vi "Register gRPC Messages.vi"(8 "error in (no error)":errorcluster, 11 "gRPC ID":T1) -> (0 "error out":errorcluster, 3 "gRPC ID Out":T1)   [LabVIEW 2021, in "NI Switch_client.lvlib"]
uses:
  NI Switch_client.lvlib
  <vilib>/gRPC/LabVIEW gRPC Library/Shared/grpcId.ctl
  <vilib>/gRPC/LabVIEW gRPC Library/Server API/typeDefs/Message Metadata.ctl
  <vilib>/gRPC/LabVIEW gRPC Library/Server API/typeDefs/Message Element Metadata.ctl
  <vilib>/gRPC/LabVIEW gRPC Library/Server API/typeDefs/Message Element Type.ctl
  <vilib>/gRPC/LabVIEW gRPC Library/Server API/typeDefs/Enum Metadata.ctl
  <vilib>/gRPC/LabVIEW gRPC Library/grpc-lvsupport-release.lvlib
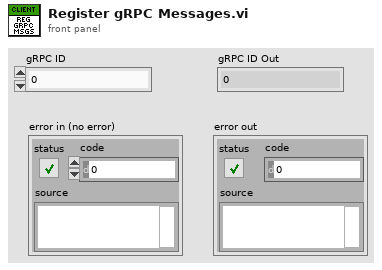
[diagram p1: front panel]
types:
  T1 = typedef "grpc-lvsupport-release.lvlib/grpcId.ctl" = u64
  T2 = typedef "grpc-lvsupport-release.lvlib/Enum Metadata.ctl" = cluster{"Version":i32, "Name":string, "Type Url":string, "Enum Values":string, "Allow Alias":bool}
  T3 = typedef "grpc-lvsupport-release.lvlib/Message Metadata.ctl" = cluster{"Version":i32, "Name":string, "Type Url":string, "Elements":T4[], "Has Oneof":bool}
  T4 = typedef "grpc-lvsupport-release.lvlib/Message Element Metadata.ctl" = cluster{"Field Name":string, "Embedded Message Name":string, "Protobuf Index":i32, "MessageElementType":T5, "Repeated":bool, "Is in Oneof":bool, "Oneof Container Name":string}
  T5 = typedef "grpc-lvsupport-release.lvlib/Message Element Type.ctl" = enum32{"Int32Value", "FloatValue", "DoubleValue", "BoolValue", "StringValue", "MessageValue", "Int64Value", "UInt32Value", "UInt64Value", "EnumValue", "Bytes", "Fixed64", "Fixed32", "SFixed64", "SFixed32", "SInt64", "SInt32"}
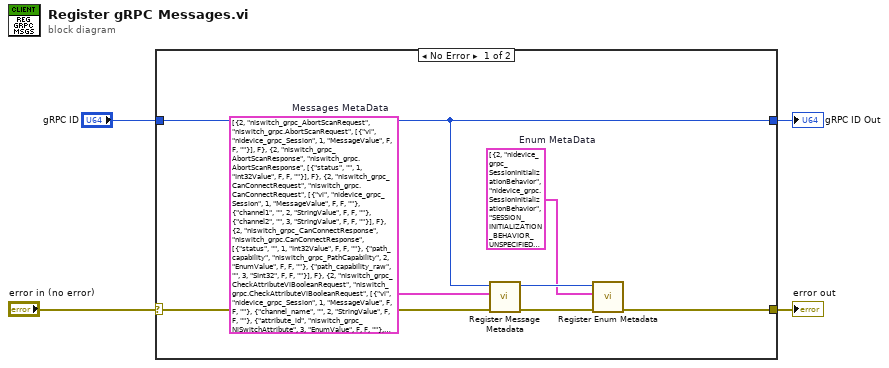
[diagram p0: block diagram]
diagram:
  n1 = case shown="No Error" "error in (no error)" {
    selector: "error in (no error)" -> [w10 w13]
    tunnel: [w9 w12] -> w1
    tunnel: [w6 w13] -> w4
    tunnel: "gRPC ID" -> [w9 w12]
    frame No Error {
      w5 = T2[] [{"Version"=2, "Name"="nidevice_grpc_SessionInitializationBehavior", "Type Url"="nidevice_grpc.SessionInitializationBehavior", "Enum Values"="SESSION_INITIALIZATION_BEHAVIOR_UNSPECIFIED=0;SESSION_INITIALIZATION_BEHAVIOR_INITIALIZE_NEW=1;SESSION_INITIALIZATION_BEHAVIOR_ATTACH_TO_EXISTING=2", "Allow Alias"=FALSE}, {"Version"=2, "Name"="niswitch_grpc_NiSwitchAttribute", "Type Url"="niswitch_grpc.NiSwitchAttribute", "Enum Values"="NISWITCH_ATTRIBUTE_UNSPECIFIED=0;NISWITCH_ATTRIBUTE_RANGE_CHECK=1050002;NISWITCH_ATTRIBUTE_QUERY_INSTRUMENT_STATUS=1050003;NISWITCH_ATTRIBUTE_CACHE=1050004;NISWITCH_ATTRIBUTE_SIMULATE=1050005;NISWITCH_ATTRIBUTE_RECORD_COERCIONS=1050006;NISWITCH_ATTRIBUTE_DRIVER_SETUP=1050007;NISWITCH_ATTRIBUTE_INTERCHANGE_CHECK=1050021;NISWITCH_ATTRIBUTE_CHANNEL_COUNT=1050203;NISWITCH_ATTRIBUTE_SPECIFIC_DRIVER_PREFIX=1050302;NISWITCH_ATTRIBUTE_IO_RESOURCE_DESCRIPTOR=1050304;NISWITCH_ATTRIBUTE_LOGICAL_NAME=1050305;NISWITCH_ATTRIBUTE_SUPPORTED_INSTRUMENT_MODELS=1050327;NISWITCH_ATTRIBUTE_GROUP_CAPABILITIES=1050401;NISWITCH_ATTRIBUTE_INSTRUMENT_FIRMWARE_REVISION=1050510;NISWITCH_ATTRIBUTE_INSTRUMENT_MANUFACTURER=1050511;NISWITCH_ATTRIBUTE_INSTRUMENT_MODEL=1050512;NISWITCH_ATTRIBUTE_SPECIFIC_DRIVER_VENDOR=1050513;NISWITCH_ATTRIBUTE_SPECIFIC_DRIVER_DESCRIPTION=1050514;NISWITCH_ATTRIBUTE_SPECIFIC_DRIVER_CLASS_SPEC_MAJOR_VERSION=1050515;NISWITCH_ATTRIBUTE_SPECIFIC_DRIVER_CLASS_SPEC_MINOR_VERSION=1050516;NISWITCH_ATTRIBUTE_SPECIFIC_DRIVER_REVISION=1050551;NISWITCH_ATTRIBUTE_SERIAL_NUMBER_I32=1150001;NISWITCH_ATTRIBUTE_IS_WAITING_FOR_TRIG=1150004;NISWITCH_ATTRIBUTE_TRIGGER_MODE=1150005;NISWITCH_ATTRIBUTE_MASTER_SLAVE_TRIGGER_BUS=1150006;NISWITCH_ATTRIBUTE_MASTER_SLAVE_SCAN_ADVANCED_BUS=1150007;NISWITCH_ATTRIBUTE_CABLED_MODULE_TRIGGER_BUS=1150008;NISWITCH_ATTRIBUTE_CABLED_MODULE_SCAN_ADVANCED_BUS=1150009;NISWITCH_ATTRIBUTE_TRIGGER_INPUT_POLARITY=1150010;NISWITCH_ATTRIBUTE_SCAN_ADVANCED_POLARITY=1150011;NISWITCH_ATTRIBUTE_PARSED_SCAN_LIST=1150012;NISWITCH_ATTRIBUTE_HANDSHAKING_INITIATION=1150013;NISWITCH_ATTRIBUTE_NUMBER_OF_RELAYS=1150014;NISWITCH_ATTRIBUTE_SERIAL_NUMBER=1150015;NISWITCH_ATTRIBUTE_DIGITAL_FILTER_ENABLE=1150016;NISWITCH_ATTRIBUTE_POWER_DOWN_LATCHING_RELAYS_AFTER_DEBOUNCE=1150017;NISWITCH_ATTRIBUTE_ANALOG_BUS_SHARING_ENABLE=1150018;NISWITCH_ATTRIBUTE_TEMPERATURE=1150019;NISWITCH_ATTRIBUTE_IS_SOURCE_CHANNEL=1250001;NISWITCH_ATTRIBUTE_IS_DEBOUNCED=1250002;NISWITCH_ATTRIBUTE_IS_CONFIGURATION_CHANNEL=1250003;NISWITCH_ATTRIBUTE_SETTLING_TIME=1250004;NISWITCH_ATTRIBUTE_BANDWIDTH=1250005;NISWITCH_ATTRIBUTE_MAX_DC_VOLTAGE=1250006;NISWITCH_ATTRIBUTE_MAX_AC_VOLTAGE=1250007;NISWITCH_ATTRIBUTE_MAX_SWITCHING_DC_CURRENT=1250008;NISWITCH_ATTRIBUTE_MAX_SWITCHING_AC_CURRENT=1250009;NISWITCH_ATTRIBUTE_MAX_CARRY_DC_CURRENT=1250010;NISWITCH_ATTRIBUTE_MAX_CARRY_AC_CURRENT=1250011;NISWITCH_ATTRIBUTE_MAX_SWITCHING_DC_POWER=1250012;NISWITCH_ATTRIBUTE_MAX_SWITCHING_AC_POWER=1250013;NISWITCH_ATTRIBUTE_MAX_CARRY_DC_POWER=1250014;NISWITCH_ATTRIBUTE_MAX_CARRY_AC_POWER=1250015;NISWITCH_ATTRIBUTE_CHARACTERISTIC_IMPEDANCE=1250016;NISWITCH_ATTRIBUTE_WIRE_MODE=1250017;NISWITCH_ATTRIBUTE_NUM_OF_ROWS=1250018;NISWITCH_ATTRIBUTE_NUM_OF_COLUMNS=1250019;NISWITCH_ATTRIBUTE_SCAN_LIST=1250020;NISWITCH_ATTRIBUTE_SCAN_MODE=1250021;NISWITCH_ATTRIBUTE_TRIGGER_INPUT=1250022;NISWITCH_ATTRIBUTE_SCAN_ADVANCED_OUTPUT=1250023;NISWITCH_ATTRIBUTE_IS_SCANNING=1250024;NISWITCH_ATTRIBUTE_SCAN_DELAY=1250025;NISWITCH_ATTRIBUTE_CONTINUOUS_SCAN=1250026", "Allow Alias"=FALSE}, {"Version"=2, "Name"="niswitch_grpc_HandshakingInitiation", "Type Url"="niswitch_grpc.HandshakingInitiation", "Enum Values"="HANDSHAKING_INITIATION_NISWITCH_VAL_MEASUREMENT_DEVICE_INITIATED=0;HANDSHAKING_INITIATION_NISWITCH_VAL_SWITCH_INITIATED=1", "Allow Alias"=FALSE}, {"Version"=2, "Name"="niswitch_grpc_NiSwitchInt32AttributeValues", "Type Url"="niswitch_grpc.NiSwitchInt32AttributeValues", "Enum Values"="NISWITCH_INT32_UNSPECIFIED=0;NISWITCH_INT32_HANDSHAKING_INITIATION_VAL_MEASUREMENT_DEVICE_INITIATED=0;NISWITCH_INT32_HANDSHAKING_INITIATION_VAL_SWITCH_INITIATED=1;NISWITCH_INT32_SCAN_ADVANCED_OUTPUT_VAL_NONE=0;NISWITCH_INT32_SCAN_ADVANCED_OUTPUT_VAL_EXTERNAL=2;NISWITCH_INT32_SCAN_ADVANCED_OUTPUT_VAL_TTL0=111;NISWITCH_INT32_SCAN_ADVANCED_OUTPUT_VAL_TTL1=112;NISWITCH_INT32_SCAN_ADVANCED_OUTPUT_VAL_TTL2=113;NISWITCH_INT32_SCAN_ADVANCED_OUTPUT_VAL_TTL3=114;NISWITCH_INT32_SCAN_ADVANCED_OUTPUT_VAL_TTL4=115;NISWITCH_INT32_SCAN_ADVANCED_OUTPUT_VAL_TTL5=116;NISWITCH_INT32_SCAN_ADVANCED_OUTPUT_VAL_TTL6=117;NISWITCH_INT32_SCAN_ADVANCED_OUTPUT_VAL_TTL7=118;NISWITCH_INT32_SCAN_ADVANCED_OUTPUT_VAL_PXI_STAR=125;NISWITCH_INT32_SCAN_ADVANCED_OUTPUT_VAL_REARCONNECTOR=1000;NISWITCH_INT32_SCAN_ADVANCED_OUTPUT_VAL_FRONTCONNECTOR=1001;NISWITCH_INT32_SCAN_ADVANCED_OUTPUT_VAL_REARCONNECTOR_MODULE1=1021;NISWITCH_INT32_SCAN_ADVANCED_OUTPUT_VAL_REARCONNECTOR_MODULE2=1022;NISWITCH_INT32_SCAN_ADVANCED_OUTPUT_VAL_REARCONNECTOR_MODULE3=1023;NISWITCH_INT32_SCAN_ADVANCED_OUTPUT_VAL_REARCONNECTOR_MODULE4=1024;NISWITCH_INT32_SCAN_ADVANCED_OUTPUT_VAL_REARCONNECTOR_MODULE5=1025;NISWITCH_INT32_SCAN_ADVANCED_OUTPUT_VAL_REARCONNECTOR_MODULE6=1026;NISWITCH_INT32_SCAN_ADVANCED_OUTPUT_VAL_REARCONNECTOR_MODULE7=1027;NISWITCH_INT32_SCAN_ADVANCED_OUTPUT_VAL_REARCONNECTOR_MODULE8=1028;NISWITCH_INT32_SCAN_ADVANCED_OUTPUT_VAL_REARCONNECTOR_MODULE9=1029;NISWITCH_INT32_SCAN_ADVANCED_OUTPUT_VAL_REARCONNECTOR_MODULE10=1030;NISWITCH_INT32_SCAN_ADVANCED_OUTPUT_VAL_REARCONNECTOR_MODULE11=1031;NISWITCH_INT32_SCAN_ADVANCED_OUTPUT_VAL_REARCONNECTOR_MODULE12=1032;NISWITCH_INT32_SCAN_ADVANCED_OUTPUT_VAL_FRONTCONNECTOR_MODULE1=1041;NISWITCH_INT32_SCAN_ADVANCED_OUTPUT_VAL_FRONTCONNECTOR_MODULE2=1042;NISWITCH_INT32_SCAN_ADVANCED_OUTPUT_VAL_FRONTCONNECTOR_MODULE3=1043;NISWITCH_INT32_SCAN_ADVANCED_OUTPUT_VAL_FRONTCONNECTOR_MODULE4=1044;NISWITCH_INT32_SCAN_ADVANCED_OUTPUT_VAL_FRONTCONNECTOR_MODULE5=1045;NISWITCH_INT32_SCAN_ADVANCED_OUTPUT_VAL_FRONTCONNECTOR_MODULE6=1046;NISWITCH_INT32_SCAN_ADVANCED_OUTPUT_VAL_FRONTCONNECTOR_MODULE7=1047;NISWITCH_INT32_SCAN_ADVANCED_OUTPUT_VAL_FRONTCONNECTOR_MODULE8=1048;NISWITCH_INT32_SCAN_ADVANCED_OUTPUT_VAL_FRONTCONNECTOR_MODULE9=1049;NISWITCH_INT32_SCAN_ADVANCED_OUTPUT_VAL_FRONTCONNECTOR_MODULE10=1050;NISWITCH_INT32_SCAN_ADVANCED_OUTPUT_VAL_FRONTCONNECTOR_MODULE11=1051;NISWITCH_INT32_SCAN_ADVANCED_OUTPUT_VAL_FRONTCONNECTOR_MODULE12=1052;NISWITCH_INT32_SCAN_ADVANCED_POLARITY_VAL_RISING_EDGE=0;NISWITCH_INT32_SCAN_ADVANCED_POLARITY_VAL_FALLING_EDGE=1;NISWITCH_INT32_SCAN_MODE_VAL_NONE=0;NISWITCH_INT32_SCAN_MODE_VAL_BREAK_BEFORE_MAKE=1;NISWITCH_INT32_SCAN_MODE_VAL_BREAK_AFTER_MAKE=2;NISWITCH_INT32_TRIGGER_INPUT_VAL_IMMEDIATE=1;NISWITCH_INT32_TRIGGER_INPUT_VAL_EXTERNAL=2;NISWITCH_INT32_TRIGGER_INPUT_VAL_SOFTWARE_TRIG=3;NISWITCH_INT32_TRIGGER_INPUT_VAL_TTL0=111;NISWITCH_INT32_TRIGGER_INPUT_VAL_TTL1=112;NISWITCH_INT32_TRIGGER_INPUT_VAL_TTL2=113;NISWITCH_INT32_TRIGGER_INPUT_VAL_TTL3=114;NISWITCH_INT32_TRIGGER_INPUT_VAL_TTL4=115;NISWITCH_INT32_TRIGGER_INPUT_VAL_TTL5=116;NISWITCH_INT32_TRIGGER_INPUT_VAL_TTL6=117;NISWITCH_INT32_TRIGGER_INPUT_VAL_TTL7=118;NISWITCH_INT32_TRIGGER_INPUT_VAL_PXI_STAR=125;NISWITCH_INT32_TRIGGER_INPUT_VAL_REARCONNECTOR=1000;NISWITCH_INT32_TRIGGER_INPUT_VAL_FRONTCONNECTOR=1001;NISWITCH_INT32_TRIGGER_INPUT_VAL_REARCONNECTOR_MODULE1=1021;NISWITCH_INT32_TRIGGER_INPUT_VAL_REARCONNECTOR_MODULE2=1022;NISWITCH_INT32_TRIGGER_INPUT_VAL_REARCONNECTOR_MODULE3=1023;NISWITCH_INT32_TRIGGER_INPUT_VAL_REARCONNECTOR_MODULE4=1024;NISWITCH_INT32_TRIGGER_INPUT_VAL_REARCONNECTOR_MODULE5=1025;NISWITCH_INT32_TRIGGER_INPUT_VAL_REARCONNECTOR_MODULE6=1026;NISWITCH_INT32_TRIGGER_INPUT_VAL_REARCONNECTOR_MODULE7=1027;NISWITCH_INT32_TRIGGER_INPUT_VAL_REARCONNECTOR_MODULE8=1028;NISWITCH_INT32_TRIGGER_INPUT_VAL_REARCONNECTOR_MODULE9=1029;NISWITCH_INT32_TRIGGER_INPUT_VAL_REARCONNECTOR_MODULE10=1030;NISWITCH_INT32_TRIGGER_INPUT_VAL_REARCONNECTOR_MODULE11=1031;NISWITCH_INT32_TRIGGER_INPUT_VAL_REARCONNECTOR_MODULE12=1032;NISWITCH_INT32_TRIGGER_INPUT_VAL_FRONTCONNECTOR_MODULE1=1041;NISWITCH_INT32_TRIGGER_INPUT_VAL_FRONTCONNECTOR_MODULE2=1042;NISWITCH_INT32_TRIGGER_INPUT_VAL_FRONTCONNECTOR_MODULE3=1043;NISWITCH_INT32_TRIGGER_INPUT_VAL_FRONTCONNECTOR_MODULE4=1044;NISWITCH_INT32_TRIGGER_INPUT_VAL_FRONTCONNECTOR_MODULE5=1045;NISWITCH_INT32_TRIGGER_INPUT_VAL_FRONTCONNECTOR_MODULE6=1046;NISWITCH_INT32_TRIGGER_INPUT_VAL_FRONTCONNECTOR_MODULE7=1047;NISWITCH_INT32_TRIGGER_INPUT_VAL_FRONTCONNECTOR_MODULE8=1048;NISWITCH_INT32_TRIGGER_INPUT_VAL_FRONTCONNECTOR_MODULE9=1049;NISWITCH_INT32_TRIGGER_INPUT_VAL_FRONTCONNECTOR_MODULE10=1050;NISWITCH_INT32_TRIGGER_INPUT_VAL_FRONTCONNECTOR_MODULE11=1051;NISWITCH_INT32_TRIGGER_INPUT_VAL_FRONTCONNECTOR_MODULE12=1052;NISWITCH_INT32_TRIGGER_INPUT_POLARITY_VAL_RISING_EDGE=0;NISWITCH_INT32_TRIGGER_INPUT_POLARITY_VAL_FALLING_EDGE=1;NISWITCH_INT32_WIRE_MODE_VAL_1_WIRE=1;NISWITCH_INT32_WIRE_MODE_VAL_2_WIRE=2;NISWITCH_INT32_WIRE_MODE_VAL_4_WIRE=4", "Allow Alias"=TRUE}, {"Version"=2, "Name"="niswitch_grpc_PathCapability", "Type Url"="niswitch_grpc.PathCapability", "Enum Values"="PATH_CAPABILITY_UNSPECIFIED=0;PATH_CAPABILITY_NISWITCH_VAL_PATH_AVAILABLE=1;PATH_CAPABILITY_NISWITCH_VAL_PATH_EXISTS=2;PATH_CAPABILITY_NISWITCH_VAL_PATH_UNSUPPORTED=3;PATH_CAPABILITY_NISWITCH_VAL_RESOURCE_IN_USE=4;PATH_CAPABILITY_NISWITCH_VAL_SOURCE_CONFLICT=5;PATH_CAPABILITY_NISWITCH_VAL_CHANNEL_NOT_AVAILABLE=6", "Allow Alias"=FALSE}, {"Version"=2, "Name"="niswitch_grpc_RelayAction", "Type Url"="niswitch_grpc.RelayAction", "Enum Values"="RELAY_ACTION_UNSPECIFIED=0;RELAY_ACTION_NISWITCH_VAL_OPEN_RELAY=20;RELAY_ACTION_NISWITCH_VAL_CLOSE_RELAY=21", "Allow Alias"=FALSE}, {"Version"=2, "Name"="niswitch_grpc_RelayPosition", "Type Url"="niswitch_grpc.RelayPosition", "Enum Values"="RELAY_POSITION_UNSPECIFIED=0;RELAY_POSITION_NISWITCH_VAL_OPEN=10;RELAY_POSITION_NISWITCH_VAL_CLOSED=11", "Allow Alias"=FALSE}, {"Version"=2, "Name"="niswitch_grpc_ScanAdvancedOutput", "Type Url"="niswitch_grpc.ScanAdvancedOutput", "Enum Values"="SCAN_ADVANCED_OUTPUT_NISWITCH_VAL_NONE=0;SCAN_ADVANCED_OUTPUT_NISWITCH_VAL_EXTERNAL=2;SCAN_ADVANCED_OUTPUT_NISWITCH_VAL_TTL0=111;SCAN_ADVANCED_OUTPUT_NISWITCH_VAL_TTL1=112;SCAN_ADVANCED_OUTPUT_NISWITCH_VAL_TTL2=113;SCAN_ADVANCED_OUTPUT_NISWITCH_VAL_TTL3=114;SCAN_ADVANCED_OUTPUT_NISWITCH_VAL_TTL4=115;SCAN_ADVANCED_OUTPUT_NISWITCH_VAL_TTL5=116;SCAN_ADVANCED_OUTPUT_NISWITCH_VAL_TTL6=117;SCAN_ADVANCED_OUTPUT_NISWITCH_VAL_TTL7=118;SCAN_ADVANCED_OUTPUT_NISWITCH_VAL_PXI_STAR=125;SCAN_ADVANCED_OUTPUT_NISWITCH_VAL_REARCONNECTOR=1000;SCAN_ADVANCED_OUTPUT_NISWITCH_VAL_FRONTCONNECTOR=1001;SCAN_ADVANCED_OUTPUT_NISWITCH_VAL_REARCONNECTOR_MODULE1=1021;SCAN_ADVANCED_OUTPUT_NISWITCH_VAL_REARCONNECTOR_MODULE2=1022;SCAN_ADVANCED_OUTPUT_NISWITCH_VAL_REARCONNECTOR_MODULE3=1023;SCAN_ADVANCED_OUTPUT_NISWITCH_VAL_REARCONNECTOR_MODULE4=1024;SCAN_ADVANCED_OUTPUT_NISWITCH_VAL_REARCONNECTOR_MODULE5=1025;SCAN_ADVANCED_OUTPUT_NISWITCH_VAL_REARCONNECTOR_MODULE6=1026;SCAN_ADVANCED_OUTPUT_NISWITCH_VAL_REARCONNECTOR_MODULE7=1027;SCAN_ADVANCED_OUTPUT_NISWITCH_VAL_REARCONNECTOR_MODULE8=1028;SCAN_ADVANCED_OUTPUT_NISWITCH_VAL_REARCONNECTOR_MODULE9=1029;SCAN_ADVANCED_OUTPUT_NISWITCH_VAL_REARCONNECTOR_MODULE10=1030;SCAN_ADVANCED_OUTPUT_NISWITCH_VAL_REARCONNECTOR_MODULE11=1031;SCAN_ADVANCED_OUTPUT_NISWITCH_VAL_REARCONNECTOR_MODULE12=1032;SCAN_ADVANCED_OUTPUT_NISWITCH_VAL_FRONTCONNECTOR_MODULE1=1041;SCAN_ADVANCED_OUTPUT_NISWITCH_VAL_FRONTCONNECTOR_MODULE2=1042;SCAN_ADVANCED_OUTPUT_NISWITCH_VAL_FRONTCONNECTOR_MODULE3=1043;SCAN_ADVANCED_OUTPUT_NISWITCH_VAL_FRONTCONNECTOR_MODULE4=1044;SCAN_ADVANCED_OUTPUT_NISWITCH_VAL_FRONTCONNECTOR_MODULE5=1045;SCAN_ADVANCED_OUTPUT_NISWITCH_VAL_FRONTCONNECTOR_MODULE6=1046;SCAN_ADVANCED_OUTPUT_NISWITCH_VAL_FRONTCONNECTOR_MODULE7=1047;SCAN_ADVANCED_OUTPUT_NISWITCH_VAL_FRONTCONNECTOR_MODULE8=1048;SCAN_ADVANCED_OUTPUT_NISWITCH_VAL_FRONTCONNECTOR_MODULE9=1049;SCAN_ADVANCED_OUTPUT_NISWITCH_VAL_FRONTCONNECTOR_MODULE10=1050;SCAN_ADVANCED_OUTPUT_NISWITCH_VAL_FRONTCONNECTOR_MODULE11=1051;SCAN_ADVANCED_OUTPUT_NISWITCH_VAL_FRONTCONNECTOR_MODULE12=1052", "Allow Alias"=FALSE}, {"Version"=2, "Name"="niswitch_grpc_ScanMode", "Type Url"="niswitch_grpc.ScanMode", "Enum Values"="SCAN_MODE_NISWITCH_VAL_NONE=0;SCAN_MODE_NISWITCH_VAL_BREAK_BEFORE_MAKE=1;SCAN_MODE_NISWITCH_VAL_BREAK_AFTER_MAKE=2", "Allow Alias"=FALSE}, {"Version"=2, "Name"="niswitch_grpc_TriggerInput", "Type Url"="niswitch_grpc.TriggerInput", "Enum Values"="TRIGGER_INPUT_UNSPECIFIED=0;TRIGGER_INPUT_NISWITCH_VAL_IMMEDIATE=1;TRIGGER_INPUT_NISWITCH_VAL_EXTERNAL=2;TRIGGER_INPUT_NISWITCH_VAL_SOFTWARE_TRIG=3;TRIGGER_INPUT_NISWITCH_VAL_TTL0=111;TRIGGER_INPUT_NISWITCH_VAL_TTL1=112;TRIGGER_INPUT_NISWITCH_VAL_TTL2=113;TRIGGER_INPUT_NISWITCH_VAL_TTL3=114;TRIGGER_INPUT_NISWITCH_VAL_TTL4=115;TRIGGER_INPUT_NISWITCH_VAL_TTL5=116;TRIGGER_INPUT_NISWITCH_VAL_TTL6=117;TRIGGER_INPUT_NISWITCH_VAL_TTL7=118;TRIGGER_INPUT_NISWITCH_VAL_PXI_STAR=125;TRIGGER_INPUT_NISWITCH_VAL_REARCONNECTOR=1000;TRIGGER_INPUT_NISWITCH_VAL_FRONTCONNECTOR=1001;TRIGGER_INPUT_NISWITCH_VAL_REARCONNECTOR_MODULE1=1021;TRIGGER_INPUT_NISWITCH_VAL_REARCONNECTOR_MODULE2=1022;TRIGGER_INPUT_NISWITCH_VAL_REARCONNECTOR_MODULE3=1023;TRIGGER_INPUT_NISWITCH_VAL_REARCONNECTOR_MODULE4=1024;TRIGGER_INPUT_NISWITCH_VAL_REARCONNECTOR_MODULE5=1025;TRIGGER_INPUT_NISWITCH_VAL_REARCONNECTOR_MODULE6=1026;TRIGGER_INPUT_NISWITCH_VAL_REARCONNECTOR_MODULE7=1027;TRIGGER_INPUT_NISWITCH_VAL_REARCONNECTOR_MODULE8=1028;TRIGGER_INPUT_NISWITCH_VAL_REARCONNECTOR_MODULE9=1029;TRIGGER_INPUT_NISWITCH_VAL_REARCONNECTOR_MODULE10=1030;TRIGGER_INPUT_NISWITCH_VAL_REARCONNECTOR_MODULE11=1031;TRIGGER_INPUT_NISWITCH_VAL_REARCONNECTOR_MODULE12=1032;TRIGGER_INPUT_NISWITCH_VAL_FRONTCONNECTOR_MODULE1=1041;TRIGGER_INPUT_NISWITCH_VAL_FRONTCONNECTOR_MODULE2=1042;TRIGGER_INPUT_NISWITCH_VAL_FRONTCONNECTOR_MODULE3=1043;TRIGGER_INPUT_NISWITCH_VAL_FRONTCONNECTOR_MODULE4=1044;TRIGGER_INPUT_NISWITCH_VAL_FRONTCONNECTOR_MODULE5=1045;TRIGGER_INPUT_NISWITCH_VAL_FRONTCONNECTOR_MODULE6=1046;TRIGGER_INPUT_NISWITCH_VAL_FRONTCONNECTOR_MODULE7=1047;TRIGGER_INPUT_NISWITCH_VAL_FRONTCONNECTOR_MODULE8=1048;TRIGGER_INPUT_NISWITCH_VAL_FRONTCONNECTOR_MODULE9=1049;TRIGGER_INPUT_NISWITCH_VAL_FRONTCONNECTOR_MODULE10=1050;TRIGGER_INPUT_NISWITCH_VAL_FRONTCONNECTOR_MODULE11=1051;TRIGGER_INPUT_NISWITCH_VAL_FRONTCONNECTOR_MODULE12=1052", "Allow Alias"=FALSE}]  # Enum MetaData
      w11 = T3[] [{"Version"=2, "Name"="niswitch_grpc_AbortScanRequest", "Type Url"="niswitch_grpc.AbortScanRequest", "Elements"=[{"Field Name"="vi", "Embedded Message Name"="nidevice_grpc_Session", "Protobuf Index"=1, "MessageElementType"=enum."MessageValue", "Repeated"=FALSE, "Is in Oneof"=FALSE, "Oneof Container Name"=""}], "Has Oneof"=FALSE}, {"Version"=2, "Name"="niswitch_grpc_AbortScanResponse", "Type Url"="niswitch_grpc.AbortScanResponse", "Elements"=[{"Field Name"="status", "Embedded Message Name"="", "Protobuf Index"=1, "MessageElementType"=enum."Int32Value", "Repeated"=FALSE, "Is in Oneof"=FALSE, "Oneof Container Name"=""}], "Has Oneof"=FALSE}, {"Version"=2, "Name"="niswitch_grpc_CanConnectRequest", "Type Url"="niswitch_grpc.CanConnectRequest", "Elements"=[{"Field Name"="vi", "Embedded Message Name"="nidevice_grpc_Session", "Protobuf Index"=1, "MessageElementType"=enum."MessageValue", "Repeated"=FALSE, "Is in Oneof"=FALSE, "Oneof Container Name"=""}, {"Field Name"="channel1", "Embedded Message Name"="", "Protobuf Index"=2, "MessageElementType"=enum."StringValue", "Repeated"=FALSE, "Is in Oneof"=FALSE, "Oneof Container Name"=""}, {"Field Name"="channel2", "Embedded Message Name"="", "Protobuf Index"=3, "MessageElementType"=enum."StringValue", "Repeated"=FALSE, "Is in Oneof"=FALSE, "Oneof Container Name"=""}], "Has Oneof"=FALSE}, {"Version"=2, "Name"="niswitch_grpc_CanConnectResponse", "Type Url"="niswitch_grpc.CanConnectResponse", "Elements"=[{"Field Name"="status", "Embedded Message Name"="", "Protobuf Index"=1, "MessageElementType"=enum."Int32Value", "Repeated"=FALSE, "Is in Oneof"=FALSE, "Oneof Container Name"=""}, {"Field Name"="path_capability", "Embedded Message Name"="niswitch_grpc_PathCapability", "Protobuf Index"=2, "MessageElementType"=enum."EnumValue", "Repeated"=FALSE, "Is in Oneof"=FALSE, "Oneof Container Name"=""}, {"Field Name"="path_capability_raw", "Embedded Message Name"="", "Protobuf Index"=3, "MessageElementType"=enum."SInt32", "Repeated"=FALSE, "Is in Oneof"=FALSE, "Oneof Container Name"=""}], "Has Oneof"=FALSE}, {"Version"=2, "Name"="niswitch_grpc_CheckAttributeViBooleanRequest", "Type Url"="niswitch_grpc.CheckAttributeViBooleanRequest", "Elements"=[{"Field Name"="vi", "Embedded Message Name"="nidevice_grpc_Session", "Protobuf Index"=1, "MessageElementType"=enum."MessageValue", "Repeated"=FALSE, "Is in Oneof"=FALSE, "Oneof Container Name"=""}, {"Field Name"="channel_name", "Embedded Message Name"="", "Protobuf Index"=2, "MessageElementType"=enum."StringValue", "Repeated"=FALSE, "Is in Oneof"=FALSE, "Oneof Container Name"=""}, {"Field Name"="attribute_id", "Embedded Message Name"="niswitch_grpc_NiSwitchAttribute", "Protobuf Index"=3, "MessageElementType"=enum."EnumValue", "Repeated"=FALSE, "Is in Oneof"=FALSE, "Oneof Container Name"=""}, {"Field Name"="attribute_value", "Embedded Message Name"="", "Protobuf Index"=4, "MessageElementType"=enum."BoolValue", "Repeated"=FALSE, "Is in Oneof"=FALSE, "Oneof Container Name"=""}], "Has Oneof"=FALSE}, {"Version"=2, "Name"="niswitch_grpc_CheckAttributeViBooleanResponse", "Type Url"="niswitch_grpc.CheckAttributeViBooleanResponse", "Elements"=[{"Field Name"="status", "Embedded Message Name"="", "Protobuf Index"=1, "MessageElementType"=enum."Int32Value", "Repeated"=FALSE, "Is in Oneof"=FALSE, "Oneof Container Name"=""}], "Has Oneof"=FALSE}, {"Version"=2, "Name"="niswitch_grpc_CheckAttributeViInt32Request", "Type Url"="niswitch_grpc.CheckAttributeViInt32Request", "Elements"=[{"Field Name"="vi", "Embedded Message Name"="nidevice_grpc_Session", "Protobuf Index"=1, "MessageElementType"=enum."MessageValue", "Repeated"=FALSE, "Is in Oneof"=FALSE, "Oneof Container Name"=""}, {"Field Name"="channel_name", "Embedded Message Name"="", "Protobuf Index"=2, "MessageElementType"=enum."StringValue", "Repeated"=FALSE, "Is in Oneof"=FALSE, "Oneof Container Name"=""}, {"Field Name"="attribute_id", "Embedded Message Name"="niswitch_grpc_NiSwitchAttribute", "Protobuf Index"=3, "MessageElementType"=enum."EnumValue", "Repeated"=FALSE, "Is in Oneof"=FALSE, "Oneof Container Name"=""}, {"Field Name"="selected_index", "Embedded Message Name"="", "Protobuf Index"=-1, "MessageElementType"=enum."Int32Value", "Repeated"=FALSE, "Is in Oneof"=TRUE, "Oneof Container Name"="niswitch_grpc_CheckAttributeViInt32Request_attribute_value_enum"}, {"Field Name"="attribute_value_raw", "Embedded Message Name"="", "Protobuf Index"=4, "MessageElementType"=enum."SInt32", "Repeated"=FALSE, "Is in Oneof"=TRUE, "Oneof Container Name"="niswitch_grpc_CheckAttributeViInt32Request_attribute_value_enum"}, {"Field Name"="attribute_value", "Embedded Message Name"="niswitch_grpc_NiSwitchInt32AttributeValues", "Protobuf Index"=5, "MessageElementType"=enum."EnumValue", "Repeated"=FALSE, "Is in Oneof"=TRUE, "Oneof Container Name"="niswitch_grpc_CheckAttributeViInt32Request_attribute_value_enum"}], "Has Oneof"=TRUE}, {"Version"=2, "Name"="niswitch_grpc_CheckAttributeViInt32Response", "Type Url"="niswitch_grpc.CheckAttributeViInt32Response", "Elements"=[{"Field Name"="status", "Embedded Message Name"="", "Protobuf Index"=1, "MessageElementType"=enum."Int32Value", "Repeated"=FALSE, "Is in Oneof"=FALSE, "Oneof Container Name"=""}], "Has Oneof"=FALSE}, {"Version"=2, "Name"="niswitch_grpc_CheckAttributeViReal64Request", "Type Url"="niswitch_grpc.CheckAttributeViReal64Request", "Elements"=[{"Field Name"="vi", "Embedded Message Name"="nidevice_grpc_Session", "Protobuf Index"=1, "MessageElementType"=enum."MessageValue", "Repeated"=FALSE, "Is in Oneof"=FALSE, "Oneof Container Name"=""}, {"Field Name"="channel_name", "Embedded Message Name"="", "Protobuf Index"=2, "MessageElementType"=enum."StringValue", "Repeated"=FALSE, "Is in Oneof"=FALSE, "Oneof Container Name"=""}, {"Field Name"="attribute_id", "Embedded Message Name"="niswitch_grpc_NiSwitchAttribute", "Protobuf Index"=3, "MessageElementType"=enum."EnumValue", "Repeated"=FALSE, "Is in Oneof"=FALSE, "Oneof Container Name"=""}, {"Field Name"="attribute_value_raw", "Embedded Message Name"="", "Protobuf Index"=4, "MessageElementType"=enum."DoubleValue", "Repeated"=FALSE, "Is in Oneof"=FALSE, "Oneof Container Name"=""}], "Has Oneof"=FALSE}, {"Version"=2, "Name"="niswitch_grpc_CheckAttributeViReal64Response", "Type Url"="niswitch_grpc.CheckAttributeViReal64Response", "Elements"=[{"Field Name"="status", "Embedded Message Name"="", "Protobuf Index"=1, "MessageElementType"=enum."Int32Value", "Repeated"=FALSE, "Is in Oneof"=FALSE, "Oneof Container Name"=""}], "Has Oneof"=FALSE}, {"Version"=2, "Name"="niswitch_grpc_CheckAttributeViSessionRequest", "Type Url"="niswitch_grpc.CheckAttributeViSessionRequest", "Elements"=[{"Field Name"="vi", "Embedded Message Name"="nidevice_grpc_Session", "Protobuf Index"=1, "MessageElementType"=enum."MessageValue", "Repeated"=FALSE, "Is in Oneof"=FALSE, "Oneof Container Name"=""}, {"Field Name"="channel_name", "Embedded Message Name"="", "Protobuf Index"=2, "MessageElementType"=enum."StringValue", "Repeated"=FALSE, "Is in Oneof"=FALSE, "Oneof Container Name"=""}, {"Field Name"="attribute_id", "Embedded Message Name"="niswitch_grpc_NiSwitchAttribute", "Protobuf Index"=3, "MessageElementType"=enum."EnumValue", "Repeated"=FALSE, "Is in Oneof"=FALSE, "Oneof Container Name"=""}, {"Field Name"="attribute_value", "Embedded Message Name"="nidevice_grpc_Session", "Protobuf Index"=4, "MessageElementType"=enum."MessageValue", "Repeated"=FALSE, "Is in Oneof"=FALSE, "Oneof Container Name"=""}], "Has Oneof"=FALSE}, {"Version"=2, "Name"="niswitch_grpc_CheckAttributeViSessionResponse", "Type Url"="niswitch_grpc.CheckAttributeViSessionResponse", "Elements"=[{"Field Name"="status", "Embedded Message Name"="", "Protobuf Index"=1, "MessageElementType"=enum."Int32Value", "Repeated"=FALSE, "Is in Oneof"=FALSE, "Oneof Container Name"=""}], "Has Oneof"=FALSE}, {"Version"=2, "Name"="niswitch_grpc_CheckAttributeViStringRequest", "Type Url"="niswitch_grpc.CheckAttributeViStringRequest", "Elements"=[{"Field Name"="vi", "Embedded Message Name"="nidevice_grpc_Session", "Protobuf Index"=1, "MessageElementType"=enum."MessageValue", "Repeated"=FALSE, "Is in Oneof"=FALSE, "Oneof Container Name"=""}, {"Field Name"="channel_name", "Embedded Message Name"="", "Protobuf Index"=2, "MessageElementType"=enum."StringValue", "Repeated"=FALSE, "Is in Oneof"=FALSE, "Oneof Container Name"=""}, {"Field Name"="attribute_id", "Embedded Message Name"="niswitch_grpc_NiSwitchAttribute", "Protobuf Index"=3, "MessageElementType"=enum."EnumValue", "Repeated"=FALSE, "Is in Oneof"=FALSE, "Oneof Container Name"=""}, {"Field Name"="attribute_value_raw", "Embedded Message Name"="", "Protobuf Index"=4, "MessageElementType"=enum."StringValue", "Repeated"=FALSE, "Is in Oneof"=FALSE, "Oneof Container Name"=""}], "Has Oneof"=FALSE}, {"Version"=2, "Name"="niswitch_grpc_CheckAttributeViStringResponse", "Type Url"="niswitch_grpc.CheckAttributeViStringResponse", "Elements"=[{"Field Name"="status", "Embedded Message Name"="", "Protobuf Index"=1, "MessageElementType"=enum."Int32Value", "Repeated"=FALSE, "Is in Oneof"=FALSE, "Oneof Container Name"=""}], "Has Oneof"=FALSE}, {"Version"=2, "Name"="niswitch_grpc_ClearErrorRequest", "Type Url"="niswitch_grpc.ClearErrorRequest", "Elements"=[{"Field Name"="vi", "Embedded Message Name"="nidevice_grpc_Session", "Protobuf Index"=1, "MessageElementType"=enum."MessageValue", "Repeated"=FALSE, "Is in Oneof"=FALSE, "Oneof Container Name"=""}], "Has Oneof"=FALSE}, {"Version"=2, "Name"="niswitch_grpc_ClearErrorResponse", "Type Url"="niswitch_grpc.ClearErrorResponse", "Elements"=[{"Field Name"="status", "Embedded Message Name"="", "Protobuf Index"=1, "MessageElementType"=enum."Int32Value", "Repeated"=FALSE, "Is in Oneof"=FALSE, "Oneof Container Name"=""}], "Has Oneof"=FALSE}, {"Version"=2, "Name"="niswitch_grpc_ClearInterchangeWarningsRequest", "Type Url"="niswitch_grpc.ClearInterchangeWarningsRequest", "Elements"=[{"Field Name"="vi", "Embedded Message Name"="nidevice_grpc_Session", "Protobuf Index"=1, "MessageElementType"=enum."MessageValue", "Repeated"=FALSE, "Is in Oneof"=FALSE, "Oneof Container Name"=""}], "Has Oneof"=FALSE}, {"Version"=2, "Name"="niswitch_grpc_ClearInterchangeWarningsResponse", "Type Url"="niswitch_grpc.ClearInterchangeWarningsResponse", "Elements"=[{"Field Name"="status", "Embedded Message Name"="", "Protobuf Index"=1, "MessageElementType"=enum."Int32Value", "Repeated"=FALSE, "Is in Oneof"=FALSE, "Oneof Container Name"=""}], "Has Oneof"=FALSE}, {"Version"=2, "Name"="niswitch_grpc_CloseRequest", "Type Url"="niswitch_grpc.CloseRequest", "Elements"=[{"Field Name"="vi", "Embedded Message Name"="nidevice_grpc_Session", "Protobuf Index"=1, "MessageElementType"=enum."MessageValue", "Repeated"=FALSE, "Is in Oneof"=FALSE, "Oneof Container Name"=""}], "Has Oneof"=FALSE}, {"Version"=2, "Name"="niswitch_grpc_CloseResponse", "Type Url"="niswitch_grpc.CloseResponse", "Elements"=[{"Field Name"="status", "Embedded Message Name"="", "Protobuf Index"=1, "MessageElementType"=enum."Int32Value", "Repeated"=FALSE, "Is in Oneof"=FALSE, "Oneof Container Name"=""}], "Has Oneof"=FALSE}, {"Version"=2, "Name"="niswitch_grpc_CommitRequest", "Type Url"="niswitch_grpc.CommitRequest", "Elements"=[{"Field Name"="vi", "Embedded Message Name"="nidevice_grpc_Session", "Protobuf Index"=1, "MessageElementType"=enum."MessageValue", "Repeated"=FALSE, "Is in Oneof"=FALSE, "Oneof Container Name"=""}], "Has Oneof"=FALSE}, {"Version"=2, "Name"="niswitch_grpc_CommitResponse", "Type Url"="niswitch_grpc.CommitResponse", "Elements"=[{"Field Name"="status", "Embedded Message Name"="", "Protobuf Index"=1, "MessageElementType"=enum."Int32Value", "Repeated"=FALSE, "Is in Oneof"=FALSE, "Oneof Container Name"=""}], "Has Oneof"=FALSE}, {"Version"=2, "Name"="niswitch_grpc_ConfigureScanListRequest", "Type Url"="niswitch_grpc.ConfigureScanListRequest", "Elements"=[{"Field Name"="vi", "Embedded Message Name"="nidevice_grpc_Session", "Protobuf Index"=1, "MessageElementType"=enum."MessageValue", "Repeated"=FALSE, "Is in Oneof"=FALSE, "Oneof Container Name"=""}, {"Field Name"="scanlist", "Embedded Message Name"="", "Protobuf Index"=2, "MessageElementType"=enum."StringValue", "Repeated"=FALSE, "Is in Oneof"=FALSE, "Oneof Container Name"=""}, {"Field Name"="selected_index", "Embedded Message Name"="", "Protobuf Index"=-1, "MessageElementType"=enum."Int32Value", "Repeated"=FALSE, "Is in Oneof"=TRUE, "Oneof Container Name"="niswitch_grpc_ConfigureScanListRequest_scan_mode_enum"}, {"Field Name"="scan_mode", "Embedded Message Name"="niswitch_grpc_ScanMode", "Protobuf Index"=3, "MessageElementType"=enum."EnumValue", "Repeated"=FALSE, "Is in Oneof"=TRUE, "Oneof Container Name"="niswitch_grpc_ConfigureScanListRequest_scan_mode_enum"}, {"Field Name"="scan_mode_raw", "Embedded Message Name"="", "Protobuf Index"=4, "MessageElementType"=enum."SInt32", "Repeated"=FALSE, "Is in Oneof"=TRUE, "Oneof Container Name"="niswitch_grpc_ConfigureScanListRequest_scan_mode_enum"}], "Has Oneof"=TRUE}, {"Version"=2, "Name"="niswitch_grpc_ConfigureScanListResponse", "Type Url"="niswitch_grpc.ConfigureScanListResponse", "Elements"=[{"Field Name"="status", "Embedded Message Name"="", "Protobuf Index"=1, "MessageElementType"=enum."Int32Value", "Repeated"=FALSE, "Is in Oneof"=FALSE, "Oneof Container Name"=""}], "Has Oneof"=FALSE}, {"Version"=2, "Name"="niswitch_grpc_ConfigureScanTriggerRequest", "Type Url"="niswitch_grpc.ConfigureScanTriggerRequest", "Elements"=[{"Field Name"="vi", "Embedded Message Name"="nidevice_grpc_Session", "Protobuf Index"=1, "MessageElementType"=enum."MessageValue", "Repeated"=FALSE, "Is in Oneof"=FALSE, "Oneof Container Name"=""}, {"Field Name"="scan_delay", "Embedded Message Name"="", "Protobuf Index"=2, "MessageElementType"=enum."DoubleValue", "Repeated"=FALSE, "Is in Oneof"=FALSE, "Oneof Container Name"=""}, {"Field Name"="selected_index", "Embedded Message Name"="", "Protobuf Index"=-1, "MessageElementType"=enum."Int32Value", "Repeated"=FALSE, "Is in Oneof"=TRUE, "Oneof Container Name"="niswitch_grpc_ConfigureScanTriggerRequest_trigger_input_enum"}, {"Field Name"="trigger_input", "Embedded Message Name"="niswitch_grpc_TriggerInput", "Protobuf Index"=3, "MessageElementType"=enum."EnumValue", "Repeated"=FALSE, "Is in Oneof"=TRUE, "Oneof Container Name"="niswitch_grpc_ConfigureScanTriggerRequest_trigger_input_enum"}, {"Field Name"="trigger_input_raw", "Embedded Message Name"="", "Protobuf Index"=4, "MessageElementType"=enum."SInt32", "Repeated"=FALSE, "Is in Oneof"=TRUE, "Oneof Container Name"="niswitch_grpc_ConfigureScanTriggerRequest_trigger_input_enum"}, {"Field Name"="selected_index", "Embedded Message Name"="", "Protobuf Index"=-1, "MessageElementType"=enum."Int32Value", "Repeated"=FALSE, "Is in Oneof"=TRUE, "Oneof Container Name"="niswitch_grpc_ConfigureScanTriggerRequest_scan_advanced_output_enum"}, {"Field Name"="scan_advanced_output", "Embedded Message Name"="niswitch_grpc_ScanAdvancedOutput", "Protobuf Index"=5, "MessageElementType"=enum."EnumValue", "Repeated"=FALSE, "Is in Oneof"=TRUE, "Oneof Container Name"="niswitch_grpc_ConfigureScanTriggerRequest_scan_advanced_output_enum"}, {"Field Name"="scan_advanced_output_raw", "Embedded Message Name"="", "Protobuf Index"=6, "MessageElementType"=enum."SInt32", "Repeated"=FALSE, "Is in Oneof"=TRUE, "Oneof Container Name"="niswitch_grpc_ConfigureScanTriggerRequest_scan_advanced_output_enum"}], "Has Oneof"=TRUE}, {"Version"=2, "Name"="niswitch_grpc_ConfigureScanTriggerResponse", "Type Url"="niswitch_grpc.ConfigureScanTriggerResponse", "Elements"=[{"Field Name"="status", "Embedded Message Name"="", "Protobuf Index"=1, "MessageElementType"=enum."Int32Value", "Repeated"=FALSE, "Is in Oneof"=FALSE, "Oneof Container Name"=""}], "Has Oneof"=FALSE}, {"Version"=2, "Name"="niswitch_grpc_ConnectRequest", "Type Url"="niswitch_grpc.ConnectRequest", "Elements"=[{"Field Name"="vi", "Embedded Message Name"="nidevice_grpc_Session", "Protobuf Index"=1, "MessageElementType"=enum."MessageValue", "Repeated"=FALSE, "Is in Oneof"=FALSE, "Oneof Container Name"=""}, {"Field Name"="channel1", "Embedded Message Name"="", "Protobuf Index"=2, "MessageElementType"=enum."StringValue", "Repeated"=FALSE, "Is in Oneof"=FALSE, "Oneof Container Name"=""}, {"Field Name"="channel2", "Embedded Message Name"="", "Protobuf Index"=3, "MessageElementType"=enum."StringValue", "Repeated"=FALSE, "Is in Oneof"=FALSE, "Oneof Container Name"=""}], "Has Oneof"=FALSE}, {"Version"=2, "Name"="niswitch_grpc_ConnectResponse", "Type Url"="niswitch_grpc.ConnectResponse", "Elements"=[{"Field Name"="status", "Embedded Message Name"="", "Protobuf Index"=1, "MessageElementType"=enum."Int32Value", "Repeated"=FALSE, "Is in Oneof"=FALSE, "Oneof Container Name"=""}], "Has Oneof"=FALSE}, {"Version"=2, "Name"="niswitch_grpc_ConnectMultipleRequest", "Type Url"="niswitch_grpc.ConnectMultipleRequest", "Elements"=[{"Field Name"="vi", "Embedded Message Name"="nidevice_grpc_Session", "Protobuf Index"=1, "MessageElementType"=enum."MessageValue", "Repeated"=FALSE, "Is in Oneof"=FALSE, "Oneof Container Name"=""}, {"Field Name"="connection_list", "Embedded Message Name"="", "Protobuf Index"=2, "MessageElementType"=enum."StringValue", "Repeated"=FALSE, "Is in Oneof"=FALSE, "Oneof Container Name"=""}], "Has Oneof"=FALSE}, {"Version"=2, "Name"="niswitch_grpc_ConnectMultipleResponse", "Type Url"="niswitch_grpc.ConnectMultipleResponse", "Elements"=[{"Field Name"="status", "Embedded Message Name"="", "Protobuf Index"=1, "MessageElementType"=enum."Int32Value", "Repeated"=FALSE, "Is in Oneof"=FALSE, "Oneof Container Name"=""}], "Has Oneof"=FALSE}, {"Version"=2, "Name"="niswitch_grpc_DisableRequest", "Type Url"="niswitch_grpc.DisableRequest", "Elements"=[{"Field Name"="vi", "Embedded Message Name"="nidevice_grpc_Session", "Protobuf Index"=1, "MessageElementType"=enum."MessageValue", "Repeated"=FALSE, "Is in Oneof"=FALSE, "Oneof Container Name"=""}], "Has Oneof"=FALSE}, {"Version"=2, "Name"="niswitch_grpc_DisableResponse", "Type Url"="niswitch_grpc.DisableResponse", "Elements"=[{"Field Name"="status", "Embedded Message Name"="", "Protobuf Index"=1, "MessageElementType"=enum."Int32Value", "Repeated"=FALSE, "Is in Oneof"=FALSE, "Oneof Container Name"=""}], "Has Oneof"=FALSE}, {"Version"=2, "Name"="niswitch_grpc_DisconnectRequest", "Type Url"="niswitch_grpc.DisconnectRequest", "Elements"=[{"Field Name"="vi", "Embedded Message Name"="nidevice_grpc_Session", "Protobuf Index"=1, "MessageElementType"=enum."MessageValue", "Repeated"=FALSE, "Is in Oneof"=FALSE, "Oneof Container Name"=""}, {"Field Name"="channel1", "Embedded Message Name"="", "Protobuf Index"=2, "MessageElementType"=enum."StringValue", "Repeated"=FALSE, "Is in Oneof"=FALSE, "Oneof Container Name"=""}, {"Field Name"="channel2", "Embedded Message Name"="", "Protobuf Index"=3, "MessageElementType"=enum."StringValue", "Repeated"=FALSE, "Is in Oneof"=FALSE, "Oneof Container Name"=""}], "Has Oneof"=FALSE}, {"Version"=2, "Name"="niswitch_grpc_DisconnectResponse", "Type Url"="niswitch_grpc.DisconnectResponse", "Elements"=[{"Field Name"="status", "Embedded Message Name"="", "Protobuf Index"=1, "MessageElementType"=enum."Int32Value", "Repeated"=FALSE, "Is in Oneof"=FALSE, "Oneof Container Name"=""}], "Has Oneof"=FALSE}, {"Version"=2, "Name"="niswitch_grpc_DisconnectAllRequest", "Type Url"="niswitch_grpc.DisconnectAllRequest", "Elements"=[{"Field Name"="vi", "Embedded Message Name"="nidevice_grpc_Session", "Protobuf Index"=1, "MessageElementType"=enum."MessageValue", "Repeated"=FALSE, "Is in Oneof"=FALSE, "Oneof Container Name"=""}], "Has Oneof"=FALSE}, {"Version"=2, "Name"="niswitch_grpc_DisconnectAllResponse", "Type Url"="niswitch_grpc.DisconnectAllResponse", "Elements"=[{"Field Name"="status", "Embedded Message Name"="", "Protobuf Index"=1, "MessageElementType"=enum."Int32Value", "Repeated"=FALSE, "Is in Oneof"=FALSE, "Oneof Container Name"=""}], "Has Oneof"=FALSE}, {"Version"=2, "Name"="niswitch_grpc_DisconnectMultipleRequest", "Type Url"="niswitch_grpc.DisconnectMultipleRequest", "Elements"=[{"Field Name"="vi", "Embedded Message Name"="nidevice_grpc_Session", "Protobuf Index"=1, "MessageElementType"=enum."MessageValue", "Repeated"=FALSE, "Is in Oneof"=FALSE, "Oneof Container Name"=""}, {"Field Name"="disconnection_list", "Embedded Message Name"="", "Protobuf Index"=2, "MessageElementType"=enum."StringValue", "Repeated"=FALSE, "Is in Oneof"=FALSE, "Oneof Container Name"=""}], "Has Oneof"=FALSE}, {"Version"=2, "Name"="niswitch_grpc_DisconnectMultipleResponse", "Type Url"="niswitch_grpc.DisconnectMultipleResponse", "Elements"=[{"Field Name"="status", "Embedded Message Name"="", "Protobuf Index"=1, "MessageElementType"=enum."Int32Value", "Repeated"=FALSE, "Is in Oneof"=FALSE, "Oneof Container Name"=""}], "Has Oneof"=FALSE}, {"Version"=2, "Name"="niswitch_grpc_ErrorMessageRequest", "Type Url"="niswitch_grpc.ErrorMessageRequest", "Elements"=[{"Field Name"="vi", "Embedded Message Name"="nidevice_grpc_Session", "Protobuf Index"=1, "MessageElementType"=enum."MessageValue", "Repeated"=FALSE, "Is in Oneof"=FALSE, "Oneof Container Name"=""}, {"Field Name"="error_code", "Embedded Message Name"="", "Protobuf Index"=2, "MessageElementType"=enum."SInt32", "Repeated"=FALSE, "Is in Oneof"=FALSE, "Oneof Container Name"=""}], "Has Oneof"=FALSE}, {"Version"=2, "Name"="niswitch_grpc_ErrorMessageResponse", "Type Url"="niswitch_grpc.ErrorMessageResponse", "Elements"=[{"Field Name"="status", "Embedded Message Name"="", "Protobuf Index"=1, "MessageElementType"=enum."Int32Value", "Repeated"=FALSE, "Is in Oneof"=FALSE, "Oneof Container Name"=""}, {"Field Name"="error_message", "Embedded Message Name"="", "Protobuf Index"=2, "MessageElementType"=enum."StringValue", "Repeated"=FALSE, "Is in Oneof"=FALSE, "Oneof Container Name"=""}], "Has Oneof"=FALSE}, {"Version"=2, "Name"="niswitch_grpc_ErrorQueryRequest", "Type Url"="niswitch_grpc.ErrorQueryRequest", "Elements"=[{"Field Name"="vi", "Embedded Message Name"="nidevice_grpc_Session", "Protobuf Index"=1, "MessageElementType"=enum."MessageValue", "Repeated"=FALSE, "Is in Oneof"=FALSE, "Oneof Container Name"=""}], "Has Oneof"=FALSE}, {"Version"=2, "Name"="niswitch_grpc_ErrorQueryResponse", "Type Url"="niswitch_grpc.ErrorQueryResponse", "Elements"=[{"Field Name"="status", "Embedded Message Name"="", "Protobuf Index"=1, "MessageElementType"=enum."Int32Value", "Repeated"=FALSE, "Is in Oneof"=FALSE, "Oneof Container Name"=""}, {"Field Name"="error_code", "Embedded Message Name"="", "Protobuf Index"=2, "MessageElementType"=enum."SInt32", "Repeated"=FALSE, "Is in Oneof"=FALSE, "Oneof Container Name"=""}, {"Field Name"="error_message", "Embedded Message Name"="", "Protobuf Index"=3, "MessageElementType"=enum."StringValue", "Repeated"=FALSE, "Is in Oneof"=FALSE, "Oneof Container Name"=""}], "Has Oneof"=FALSE}, {"Version"=2, "Name"="niswitch_grpc_GetAttributeViBooleanRequest", "Type Url"="niswitch_grpc.GetAttributeViBooleanRequest", "Elements"=[{"Field Name"="vi", "Embedded Message Name"="nidevice_grpc_Session", "Protobuf Index"=1, "MessageElementType"=enum."MessageValue", "Repeated"=FALSE, "Is in Oneof"=FALSE, "Oneof Container Name"=""}, {"Field Name"="channel_name", "Embedded Message Name"="", "Protobuf Index"=2, "MessageElementType"=enum."StringValue", "Repeated"=FALSE, "Is in Oneof"=FALSE, "Oneof Container Name"=""}, {"Field Name"="attribute_id", "Embedded Message Name"="niswitch_grpc_NiSwitchAttribute", "Protobuf Index"=3, "MessageElementType"=enum."EnumValue", "Repeated"=FALSE, "Is in Oneof"=FALSE, "Oneof Container Name"=""}], "Has Oneof"=FALSE}, {"Version"=2, "Name"="niswitch_grpc_GetAttributeViBooleanResponse", "Type Url"="niswitch_grpc.GetAttributeViBooleanResponse", "Elements"=[{"Field Name"="status", "Embedded Message Name"="", "Protobuf Index"=1, "MessageElementType"=enum."Int32Value", "Repeated"=FALSE, "Is in Oneof"=FALSE, "Oneof Container Name"=""}, {"Field Name"="attribute_value", "Embedded Message Name"="", "Protobuf Index"=2, "MessageElementType"=enum."BoolValue", "Repeated"=FALSE, "Is in Oneof"=FALSE, "Oneof Container Name"=""}], "Has Oneof"=FALSE}, {"Version"=2, "Name"="niswitch_grpc_GetAttributeViInt32Request", "Type Url"="niswitch_grpc.GetAttributeViInt32Request", "Elements"=[{"Field Name"="vi", "Embedded Message Name"="nidevice_grpc_Session", "Protobuf Index"=1, "MessageElementType"=enum."MessageValue", "Repeated"=FALSE, "Is in Oneof"=FALSE, "Oneof Container Name"=""}, {"Field Name"="channel_name", "Embedded Message Name"="", "Protobuf Index"=2, "MessageElementType"=enum."StringValue", "Repeated"=FALSE, "Is in Oneof"=FALSE, "Oneof Container Name"=""}, {"Field Name"="attribute_id", "Embedded Message Name"="niswitch_grpc_NiSwitchAttribute", "Protobuf Index"=3, "MessageElementType"=enum."EnumValue", "Repeated"=FALSE, "Is in Oneof"=FALSE, "Oneof Container Name"=""}], "Has Oneof"=FALSE}, {"Version"=2, "Name"="niswitch_grpc_GetAttributeViInt32Response", "Type Url"="niswitch_grpc.GetAttributeViInt32Response", "Elements"=[{"Field Name"="status", "Embedded Message Name"="", "Protobuf Index"=1, "MessageElementType"=enum."Int32Value", "Repeated"=FALSE, "Is in Oneof"=FALSE, "Oneof Container Name"=""}, {"Field Name"="attribute_value", "Embedded Message Name"="", "Protobuf Index"=2, "MessageElementType"=enum."SInt32", "Repeated"=FALSE, "Is in Oneof"=FALSE, "Oneof Container Name"=""}], "Has Oneof"=FALSE}, {"Version"=2, "Name"="niswitch_grpc_GetAttributeViReal64Request", "Type Url"="niswitch_grpc.GetAttributeViReal64Request", "Elements"=[{"Field Name"="vi", "Embedded Message Name"="nidevice_grpc_Session", "Protobuf Index"=1, "MessageElementType"=enum."MessageValue", "Repeated"=FALSE, "Is in Oneof"=FALSE, "Oneof Container Name"=""}, {"Field Name"="channel_name", "Embedded Message Name"="", "Protobuf Index"=2, "MessageElementType"=enum."StringValue", "Repeated"=FALSE, "Is in Oneof"=FALSE, "Oneof Container Name"=""}, {"Field Name"="attribute_id", "Embedded Message Name"="niswitch_grpc_NiSwitchAttribute", "Protobuf Index"=3, "MessageElementType"=enum."EnumValue", "Repeated"=FALSE, "Is in Oneof"=FALSE, "Oneof Container Name"=""}], "Has Oneof"=FALSE}, {"Version"=2, "Name"="niswitch_grpc_GetAttributeViReal64Response", "Type Url"="niswitch_grpc.GetAttributeViReal64Response", "Elements"=[{"Field Name"="status", "Embedded Message Name"="", "Protobuf Index"=1, "MessageElementType"=enum."Int32Value", "Repeated"=FALSE, "Is in Oneof"=FALSE, "Oneof Container Name"=""}, {"Field Name"="attribute_value", "Embedded Message Name"="", "Protobuf Index"=2, "MessageElementType"=enum."DoubleValue", "Repeated"=FALSE, "Is in Oneof"=FALSE, "Oneof Container Name"=""}], "Has Oneof"=FALSE}, {"Version"=2, "Name"="niswitch_grpc_GetAttributeViSessionRequest", "Type Url"="niswitch_grpc.GetAttributeViSessionRequest", "Elements"=[{"Field Name"="vi", "Embedded Message Name"="nidevice_grpc_Session", "Protobuf Index"=1, "MessageElementType"=enum."MessageValue", "Repeated"=FALSE, "Is in Oneof"=FALSE, "Oneof Container Name"=""}, {"Field Name"="channel_name", "Embedded Message Name"="", "Protobuf Index"=2, "MessageElementType"=enum."StringValue", "Repeated"=FALSE, "Is in Oneof"=FALSE, "Oneof Container Name"=""}, {"Field Name"="attribute_id", "Embedded Message Name"="niswitch_grpc_NiSwitchAttribute", "Protobuf Index"=3, "MessageElementType"=enum."EnumValue", "Repeated"=FALSE, "Is in Oneof"=FALSE, "Oneof Container Name"=""}], "Has Oneof"=FALSE}, {"Version"=2, "Name"="niswitch_grpc_GetAttributeViSessionResponse", "Type Url"="niswitch_grpc.GetAttributeViSessionResponse", "Elements"=[{"Field Name"="status", "Embedded Message Name"="", "Protobuf Index"=1, "MessageElementType"=enum."Int32Value", "Repeated"=FALSE, "Is in Oneof"=FALSE, "Oneof Container Name"=""}, {"Field Name"="attribute_value", "Embedded Message Name"="nidevice_grpc_Session", "Protobuf Index"=2, "MessageElementType"=enum."MessageValue", "Repeated"=FALSE, "Is in Oneof"=FALSE, "Oneof Container Name"=""}], "Has Oneof"=FALSE}, {"Version"=2, "Name"="niswitch_grpc_GetAttributeViStringRequest", "Type Url"="niswitch_grpc.GetAttributeViStringRequest", "Elements"=[{"Field Name"="vi", "Embedded Message Name"="nidevice_grpc_Session", "Protobuf Index"=1, "MessageElementType"=enum."MessageValue", "Repeated"=FALSE, "Is in Oneof"=FALSE, "Oneof Container Name"=""}, {"Field Name"="channel_name", "Embedded Message Name"="", "Protobuf Index"=2, "MessageElementType"=enum."StringValue", "Repeated"=FALSE, "Is in Oneof"=FALSE, "Oneof Container Name"=""}, {"Field Name"="attribute_id", "Embedded Message Name"="niswitch_grpc_NiSwitchAttribute", "Protobuf Index"=3, "MessageElementType"=enum."EnumValue", "Repeated"=FALSE, "Is in Oneof"=FALSE, "Oneof Container Name"=""}], "Has Oneof"=FALSE}, {"Version"=2, "Name"="niswitch_grpc_GetAttributeViStringResponse", "Type Url"="niswitch_grpc.GetAttributeViStringResponse", "Elements"=[{"Field Name"="status", "Embedded Message Name"="", "Protobuf Index"=1, "MessageElementType"=enum."Int32Value", "Repeated"=FALSE, "Is in Oneof"=FALSE, "Oneof Container Name"=""}, {"Field Name"="attribute_value", "Embedded Message Name"="", "Protobuf Index"=2, "MessageElementType"=enum."StringValue", "Repeated"=FALSE, "Is in Oneof"=FALSE, "Oneof Container Name"=""}], "Has Oneof"=FALSE}, {"Version"=2, "Name"="niswitch_grpc_GetChannelNameRequest", "Type Url"="niswitch_grpc.GetChannelNameRequest", "Elements"=[{"Field Name"="vi", "Embedded Message Name"="nidevice_grpc_Session", "Protobuf Index"=1, "MessageElementType"=enum."MessageValue", "Repeated"=FALSE, "Is in Oneof"=FALSE, "Oneof Container Name"=""}, {"Field Name"="index", "Embedded Message Name"="", "Protobuf Index"=2, "MessageElementType"=enum."SInt32", "Repeated"=FALSE, "Is in Oneof"=FALSE, "Oneof Container Name"=""}], "Has Oneof"=FALSE}, {"Version"=2, "Name"="niswitch_grpc_GetChannelNameResponse", "Type Url"="niswitch_grpc.GetChannelNameResponse", "Elements"=[{"Field Name"="status", "Embedded Message Name"="", "Protobuf Index"=1, "MessageElementType"=enum."Int32Value", "Repeated"=FALSE, "Is in Oneof"=FALSE, "Oneof Container Name"=""}, {"Field Name"="channel_name_buffer", "Embedded Message Name"="", "Protobuf Index"=2, "MessageElementType"=enum."StringValue", "Repeated"=FALSE, "Is in Oneof"=FALSE, "Oneof Container Name"=""}], "Has Oneof"=FALSE}, {"Version"=2, "Name"="niswitch_grpc_GetErrorRequest", "Type Url"="niswitch_grpc.GetErrorRequest", "Elements"=[{"Field Name"="vi", "Embedded Message Name"="nidevice_grpc_Session", "Protobuf Index"=1, "MessageElementType"=enum."MessageValue", "Repeated"=FALSE, "Is in Oneof"=FALSE, "Oneof Container Name"=""}], "Has Oneof"=FALSE}, {"Version"=2, "Name"="niswitch_grpc_GetErrorResponse", "Type Url"="niswitch_grpc.GetErrorResponse", "Elements"=[{"Field Name"="status", "Embedded Message Name"="", "Protobuf Index"=1, "MessageElementType"=enum."Int32Value", "Repeated"=FALSE, "Is in Oneof"=FALSE, "Oneof Container Name"=""}, {"Field Name"="code", "Embedded Message Name"="", "Protobuf Index"=2, "MessageElementType"=enum."SInt32", "Repeated"=FALSE, "Is in Oneof"=FALSE, "Oneof Container Name"=""}, {"Field Name"="description", "Embedded Message Name"="", "Protobuf Index"=3, "MessageElementType"=enum."StringValue", "Repeated"=FALSE, "Is in Oneof"=FALSE, "Oneof Container Name"=""}], "Has Oneof"=FALSE}, {"Version"=2, "Name"="niswitch_grpc_GetNextCoercionRecordRequest", "Type Url"="niswitch_grpc.GetNextCoercionRecordRequest", "Elements"=[{"Field Name"="vi", "Embedded Message Name"="nidevice_grpc_Session", "Protobuf Index"=1, "MessageElementType"=enum."MessageValue", "Repeated"=FALSE, "Is in Oneof"=FALSE, "Oneof Container Name"=""}], "Has Oneof"=FALSE}, {"Version"=2, "Name"="niswitch_grpc_GetNextCoercionRecordResponse", "Type Url"="niswitch_grpc.GetNextCoercionRecordResponse", "Elements"=[{"Field Name"="status", "Embedded Message Name"="", "Protobuf Index"=1, "MessageElementType"=enum."Int32Value", "Repeated"=FALSE, "Is in Oneof"=FALSE, "Oneof Container Name"=""}, {"Field Name"="coercion_record", "Embedded Message Name"="", "Protobuf Index"=2, "MessageElementType"=enum."StringValue", "Repeated"=FALSE, "Is in Oneof"=FALSE, "Oneof Container Name"=""}], "Has Oneof"=FALSE}, {"Version"=2, "Name"="niswitch_grpc_GetNextInterchangeWarningRequest", "Type Url"="niswitch_grpc.GetNextInterchangeWarningRequest", "Elements"=[{"Field Name"="vi", "Embedded Message Name"="nidevice_grpc_Session", "Protobuf Index"=1, "MessageElementType"=enum."MessageValue", "Repeated"=FALSE, "Is in Oneof"=FALSE, "Oneof Container Name"=""}], "Has Oneof"=FALSE}, {"Version"=2, "Name"="niswitch_grpc_GetNextInterchangeWarningResponse", "Type Url"="niswitch_grpc.GetNextInterchangeWarningResponse", "Elements"=[{"Field Name"="status", "Embedded Message Name"="", "Protobuf Index"=1, "MessageElementType"=enum."Int32Value", "Repeated"=FALSE, "Is in Oneof"=FALSE, "Oneof Container Name"=""}, {"Field Name"="interchange_warning", "Embedded Message Name"="", "Protobuf Index"=2, "MessageElementType"=enum."StringValue", "Repeated"=FALSE, "Is in Oneof"=FALSE, "Oneof Container Name"=""}], "Has Oneof"=FALSE}, {"Version"=2, "Name"="niswitch_grpc_GetPathRequest", "Type Url"="niswitch_grpc.GetPathRequest", "Elements"=[{"Field Name"="vi", "Embedded Message Name"="nidevice_grpc_Session", "Protobuf Index"=1, "MessageElementType"=enum."MessageValue", "Repeated"=FALSE, "Is in Oneof"=FALSE, "Oneof Container Name"=""}, {"Field Name"="channel1", "Embedded Message Name"="", "Protobuf Index"=2, "MessageElementType"=enum."StringValue", "Repeated"=FALSE, "Is in Oneof"=FALSE, "Oneof Container Name"=""}, {"Field Name"="channel2", "Embedded Message Name"="", "Protobuf Index"=3, "MessageElementType"=enum."StringValue", "Repeated"=FALSE, "Is in Oneof"=FALSE, "Oneof Container Name"=""}], "Has Oneof"=FALSE}, {"Version"=2, "Name"="niswitch_grpc_GetPathResponse", "Type Url"="niswitch_grpc.GetPathResponse", "Elements"=[{"Field Name"="status", "Embedded Message Name"="", "Protobuf Index"=1, "MessageElementType"=enum."Int32Value", "Repeated"=FALSE, "Is in Oneof"=FALSE, "Oneof Container Name"=""}, {"Field Name"="path", "Embedded Message Name"="", "Protobuf Index"=2, "MessageElementType"=enum."StringValue", "Repeated"=FALSE, "Is in Oneof"=FALSE, "Oneof Container Name"=""}], "Has Oneof"=FALSE}, {"Version"=2, "Name"="niswitch_grpc_GetRelayCountRequest", "Type Url"="niswitch_grpc.GetRelayCountRequest", "Elements"=[{"Field Name"="vi", "Embedded Message Name"="nidevice_grpc_Session", "Protobuf Index"=1, "MessageElementType"=enum."MessageValue", "Repeated"=FALSE, "Is in Oneof"=FALSE, "Oneof Container Name"=""}, {"Field Name"="relay_name", "Embedded Message Name"="", "Protobuf Index"=2, "MessageElementType"=enum."StringValue", "Repeated"=FALSE, "Is in Oneof"=FALSE, "Oneof Container Name"=""}], "Has Oneof"=FALSE}, {"Version"=2, "Name"="niswitch_grpc_GetRelayCountResponse", "Type Url"="niswitch_grpc.GetRelayCountResponse", "Elements"=[{"Field Name"="status", "Embedded Message Name"="", "Protobuf Index"=1, "MessageElementType"=enum."Int32Value", "Repeated"=FALSE, "Is in Oneof"=FALSE, "Oneof Container Name"=""}, {"Field Name"="relay_count", "Embedded Message Name"="", "Protobuf Index"=2, "MessageElementType"=enum."SInt32", "Repeated"=FALSE, "Is in Oneof"=FALSE, "Oneof Container Name"=""}], "Has Oneof"=FALSE}, {"Version"=2, "Name"="niswitch_grpc_GetRelayNameRequest", "Type Url"="niswitch_grpc.GetRelayNameRequest", "Elements"=[{"Field Name"="vi", "Embedded Message Name"="nidevice_grpc_Session", "Protobuf Index"=1, "MessageElementType"=enum."MessageValue", "Repeated"=FALSE, "Is in Oneof"=FALSE, "Oneof Container Name"=""}, {"Field Name"="index", "Embedded Message Name"="", "Protobuf Index"=2, "MessageElementType"=enum."SInt32", "Repeated"=FALSE, "Is in Oneof"=FALSE, "Oneof Container Name"=""}], "Has Oneof"=FALSE}, {"Version"=2, "Name"="niswitch_grpc_GetRelayNameResponse", "Type Url"="niswitch_grpc.GetRelayNameResponse", "Elements"=[{"Field Name"="status", "Embedded Message Name"="", "Protobuf Index"=1, "MessageElementType"=enum."Int32Value", "Repeated"=FALSE, "Is in Oneof"=FALSE, "Oneof Container Name"=""}, {"Field Name"="relay_name_buffer", "Embedded Message Name"="", "Protobuf Index"=2, "MessageElementType"=enum."StringValue", "Repeated"=FALSE, "Is in Oneof"=FALSE, "Oneof Container Name"=""}], "Has Oneof"=FALSE}, {"Version"=2, "Name"="niswitch_grpc_GetRelayPositionRequest", "Type Url"="niswitch_grpc.GetRelayPositionRequest", "Elements"=[{"Field Name"="vi", "Embedded Message Name"="nidevice_grpc_Session", "Protobuf Index"=1, "MessageElementType"=enum."MessageValue", "Repeated"=FALSE, "Is in Oneof"=FALSE, "Oneof Container Name"=""}, {"Field Name"="relay_name", "Embedded Message Name"="", "Protobuf Index"=2, "MessageElementType"=enum."StringValue", "Repeated"=FALSE, "Is in Oneof"=FALSE, "Oneof Container Name"=""}], "Has Oneof"=FALSE}, {"Version"=2, "Name"="niswitch_grpc_GetRelayPositionResponse", "Type Url"="niswitch_grpc.GetRelayPositionResponse", "Elements"=[{"Field Name"="status", "Embedded Message Name"="", "Protobuf Index"=1, "MessageElementType"=enum."Int32Value", "Repeated"=FALSE, "Is in Oneof"=FALSE, "Oneof Container Name"=""}, {"Field Name"="relay_position", "Embedded Message Name"="niswitch_grpc_RelayPosition", "Protobuf Index"=2, "MessageElementType"=enum."EnumValue", "Repeated"=FALSE, "Is in Oneof"=FALSE, "Oneof Container Name"=""}, {"Field Name"="relay_position_raw", "Embedded Message Name"="", "Protobuf Index"=3, "MessageElementType"=enum."SInt32", "Repeated"=FALSE, "Is in Oneof"=FALSE, "Oneof Container Name"=""}], "Has Oneof"=FALSE}, {"Version"=2, "Name"="niswitch_grpc_InitRequest", "Type Url"="niswitch_grpc.InitRequest", "Elements"=[{"Field Name"="session_name", "Embedded Message Name"="", "Protobuf Index"=1, "MessageElementType"=enum."StringValue", "Repeated"=FALSE, "Is in Oneof"=FALSE, "Oneof Container Name"=""}, {"Field Name"="resource_name", "Embedded Message Name"="", "Protobuf Index"=2, "MessageElementType"=enum."StringValue", "Repeated"=FALSE, "Is in Oneof"=FALSE, "Oneof Container Name"=""}, {"Field Name"="id_query", "Embedded Message Name"="", "Protobuf Index"=3, "MessageElementType"=enum."BoolValue", "Repeated"=FALSE, "Is in Oneof"=FALSE, "Oneof Container Name"=""}, {"Field Name"="reset_device", "Embedded Message Name"="", "Protobuf Index"=4, "MessageElementType"=enum."BoolValue", "Repeated"=FALSE, "Is in Oneof"=FALSE, "Oneof Container Name"=""}, {"Field Name"="initialization_behavior", "Embedded Message Name"="nidevice_grpc_SessionInitializationBehavior", "Protobuf Index"=5, "MessageElementType"=enum."EnumValue", "Repeated"=FALSE, "Is in Oneof"=FALSE, "Oneof Container Name"=""}], "Has Oneof"=FALSE}, {"Version"=2, "Name"="niswitch_grpc_InitResponse", "Type Url"="niswitch_grpc.InitResponse", "Elements"=[{"Field Name"="status", "Embedded Message Name"="", "Protobuf Index"=1, "MessageElementType"=enum."Int32Value", "Repeated"=FALSE, "Is in Oneof"=FALSE, "Oneof Container Name"=""}, {"Field Name"="vi", "Embedded Message Name"="nidevice_grpc_Session", "Protobuf Index"=2, "MessageElementType"=enum."MessageValue", "Repeated"=FALSE, "Is in Oneof"=FALSE, "Oneof Container Name"=""}, {"Field Name"="error_message", "Embedded Message Name"="", "Protobuf Index"=3, "MessageElementType"=enum."StringValue", "Repeated"=FALSE, "Is in Oneof"=FALSE, "Oneof Container Name"=""}, {"Field Name"="new_session_initialized", "Embedded Message Name"="", "Protobuf Index"=4, "MessageElementType"=enum."BoolValue", "Repeated"=FALSE, "Is in Oneof"=FALSE, "Oneof Container Name"=""}], "Has Oneof"=FALSE}, {"Version"=2, "Name"="niswitch_grpc_InitWithOptionsRequest", "Type Url"="niswitch_grpc.InitWithOptionsRequest", "Elements"=[{"Field Name"="session_name", "Embedded Message Name"="", "Protobuf Index"=1, "MessageElementType"=enum."StringValue", "Repeated"=FALSE, "Is in Oneof"=FALSE, "Oneof Container Name"=""}, {"Field Name"="resource_name", "Embedded Message Name"="", "Protobuf Index"=2, "MessageElementType"=enum."StringValue", "Repeated"=FALSE, "Is in Oneof"=FALSE, "Oneof Container Name"=""}, {"Field Name"="id_query", "Embedded Message Name"="", "Protobuf Index"=3, "MessageElementType"=enum."BoolValue", "Repeated"=FALSE, "Is in Oneof"=FALSE, "Oneof Container Name"=""}, {"Field Name"="reset_device", "Embedded Message Name"="", "Protobuf Index"=4, "MessageElementType"=enum."BoolValue", "Repeated"=FALSE, "Is in Oneof"=FALSE, "Oneof Container Name"=""}, {"Field Name"="option_string", "Embedded Message Name"="", "Protobuf Index"=5, "MessageElementType"=enum."StringValue", "Repeated"=FALSE, "Is in Oneof"=FALSE, "Oneof Container Name"=""}, {"Field Name"="initialization_behavior", "Embedded Message Name"="nidevice_grpc_SessionInitializationBehavior", "Protobuf Index"=6, "MessageElementType"=enum."EnumValue", "Repeated"=FALSE, "Is in Oneof"=FALSE, "Oneof Container Name"=""}], "Has Oneof"=FALSE}, {"Version"=2, "Name"="niswitch_grpc_InitWithOptionsResponse", "Type Url"="niswitch_grpc.InitWithOptionsResponse", "Elements"=[{"Field Name"="status", "Embedded Message Name"="", "Protobuf Index"=1, "MessageElementType"=enum."Int32Value", "Repeated"=FALSE, "Is in Oneof"=FALSE, "Oneof Container Name"=""}, {"Field Name"="vi", "Embedded Message Name"="nidevice_grpc_Session", "Protobuf Index"=2, "MessageElementType"=enum."MessageValue", "Repeated"=FALSE, "Is in Oneof"=FALSE, "Oneof Container Name"=""}, {"Field Name"="error_message", "Embedded Message Name"="", "Protobuf Index"=3, "MessageElementType"=enum."StringValue", "Repeated"=FALSE, "Is in Oneof"=FALSE, "Oneof Container Name"=""}, {"Field Name"="new_session_initialized", "Embedded Message Name"="", "Protobuf Index"=4, "MessageElementType"=enum."BoolValue", "Repeated"=FALSE, "Is in Oneof"=FALSE, "Oneof Container Name"=""}], "Has Oneof"=FALSE}, {"Version"=2, "Name"="niswitch_grpc_InitWithTopologyRequest", "Type Url"="niswitch_grpc.InitWithTopologyRequest", "Elements"=[{"Field Name"="session_name", "Embedded Message Name"="", "Protobuf Index"=1, "MessageElementType"=enum."StringValue", "Repeated"=FALSE, "Is in Oneof"=FALSE, "Oneof Container Name"=""}, {"Field Name"="resource_name", "Embedded Message Name"="", "Protobuf Index"=2, "MessageElementType"=enum."StringValue", "Repeated"=FALSE, "Is in Oneof"=FALSE, "Oneof Container Name"=""}, {"Field Name"="topology", "Embedded Message Name"="", "Protobuf Index"=3, "MessageElementType"=enum."StringValue", "Repeated"=FALSE, "Is in Oneof"=FALSE, "Oneof Container Name"=""}, {"Field Name"="simulate", "Embedded Message Name"="", "Protobuf Index"=4, "MessageElementType"=enum."BoolValue", "Repeated"=FALSE, "Is in Oneof"=FALSE, "Oneof Container Name"=""}, {"Field Name"="reset_device", "Embedded Message Name"="", "Protobuf Index"=5, "MessageElementType"=enum."BoolValue", "Repeated"=FALSE, "Is in Oneof"=FALSE, "Oneof Container Name"=""}, {"Field Name"="initialization_behavior", "Embedded Message Name"="nidevice_grpc_SessionInitializationBehavior", "Protobuf Index"=6, "MessageElementType"=enum."EnumValue", "Repeated"=FALSE, "Is in Oneof"=FALSE, "Oneof Container Name"=""}], "Has Oneof"=FALSE}, {"Version"=2, "Name"="niswitch_grpc_InitWithTopologyResponse", "Type Url"="niswitch_grpc.InitWithTopologyResponse", "Elements"=[{"Field Name"="status", "Embedded Message Name"="", "Protobuf Index"=1, "MessageElementType"=enum."Int32Value", "Repeated"=FALSE, "Is in Oneof"=FALSE, "Oneof Container Name"=""}, {"Field Name"="vi", "Embedded Message Name"="nidevice_grpc_Session", "Protobuf Index"=2, "MessageElementType"=enum."MessageValue", "Repeated"=FALSE, "Is in Oneof"=FALSE, "Oneof Container Name"=""}, {"Field Name"="error_message", "Embedded Message Name"="", "Protobuf Index"=3, "MessageElementType"=enum."StringValue", "Repeated"=FALSE, "Is in Oneof"=FALSE, "Oneof Container Name"=""}, {"Field Name"="new_session_initialized", "Embedded Message Name"="", "Protobuf Index"=4, "MessageElementType"=enum."BoolValue", "Repeated"=FALSE, "Is in Oneof"=FALSE, "Oneof Container Name"=""}], "Has Oneof"=FALSE}, {"Version"=2, "Name"="niswitch_grpc_InitiateScanRequest", "Type Url"="niswitch_grpc.InitiateScanRequest", "Elements"=[{"Field Name"="vi", "Embedded Message Name"="nidevice_grpc_Session", "Protobuf Index"=1, "MessageElementType"=enum."MessageValue", "Repeated"=FALSE, "Is in Oneof"=FALSE, "Oneof Container Name"=""}], "Has Oneof"=FALSE}, {"Version"=2, "Name"="niswitch_grpc_InitiateScanResponse", "Type Url"="niswitch_grpc.InitiateScanResponse", "Elements"=[{"Field Name"="status", "Embedded Message Name"="", "Protobuf Index"=1, "MessageElementType"=enum."Int32Value", "Repeated"=FALSE, "Is in Oneof"=FALSE, "Oneof Container Name"=""}], "Has Oneof"=FALSE}, {"Version"=2, "Name"="niswitch_grpc_InvalidateAllAttributesRequest", "Type Url"="niswitch_grpc.InvalidateAllAttributesRequest", "Elements"=[{"Field Name"="vi", "Embedded Message Name"="nidevice_grpc_Session", "Protobuf Index"=1, "MessageElementType"=enum."MessageValue", "Repeated"=FALSE, "Is in Oneof"=FALSE, "Oneof Container Name"=""}], "Has Oneof"=FALSE}, {"Version"=2, "Name"="niswitch_grpc_InvalidateAllAttributesResponse", "Type Url"="niswitch_grpc.InvalidateAllAttributesResponse", "Elements"=[{"Field Name"="status", "Embedded Message Name"="", "Protobuf Index"=1, "MessageElementType"=enum."Int32Value", "Repeated"=FALSE, "Is in Oneof"=FALSE, "Oneof Container Name"=""}], "Has Oneof"=FALSE}, {"Version"=2, "Name"="niswitch_grpc_IsDebouncedRequest", "Type Url"="niswitch_grpc.IsDebouncedRequest", "Elements"=[{"Field Name"="vi", "Embedded Message Name"="nidevice_grpc_Session", "Protobuf Index"=1, "MessageElementType"=enum."MessageValue", "Repeated"=FALSE, "Is in Oneof"=FALSE, "Oneof Container Name"=""}], "Has Oneof"=FALSE}, {"Version"=2, "Name"="niswitch_grpc_IsDebouncedResponse", "Type Url"="niswitch_grpc.IsDebouncedResponse", "Elements"=[{"Field Name"="status", "Embedded Message Name"="", "Protobuf Index"=1, "MessageElementType"=enum."Int32Value", "Repeated"=FALSE, "Is in Oneof"=FALSE, "Oneof Container Name"=""}, {"Field Name"="is_debounced", "Embedded Message Name"="", "Protobuf Index"=2, "MessageElementType"=enum."BoolValue", "Repeated"=FALSE, "Is in Oneof"=FALSE, "Oneof Container Name"=""}], "Has Oneof"=FALSE}, {"Version"=2, "Name"="niswitch_grpc_IsScanningRequest", "Type Url"="niswitch_grpc.IsScanningRequest", "Elements"=[{"Field Name"="vi", "Embedded Message Name"="nidevice_grpc_Session", "Protobuf Index"=1, "MessageElementType"=enum."MessageValue", "Repeated"=FALSE, "Is in Oneof"=FALSE, "Oneof Container Name"=""}], "Has Oneof"=FALSE}, {"Version"=2, "Name"="niswitch_grpc_IsScanningResponse", "Type Url"="niswitch_grpc.IsScanningResponse", "Elements"=[{"Field Name"="status", "Embedded Message Name"="", "Protobuf Index"=1, "MessageElementType"=enum."Int32Value", "Repeated"=FALSE, "Is in Oneof"=FALSE, "Oneof Container Name"=""}, {"Field Name"="is_scanning", "Embedded Message Name"="", "Protobuf Index"=2, "MessageElementType"=enum."BoolValue", "Repeated"=FALSE, "Is in Oneof"=FALSE, "Oneof Container Name"=""}], "Has Oneof"=FALSE}, {"Version"=2, "Name"="niswitch_grpc_RelayControlRequest", "Type Url"="niswitch_grpc.RelayControlRequest", "Elements"=[{"Field Name"="vi", "Embedded Message Name"="nidevice_grpc_Session", "Protobuf Index"=1, "MessageElementType"=enum."MessageValue", "Repeated"=FALSE, "Is in Oneof"=FALSE, "Oneof Container Name"=""}, {"Field Name"="relay_name", "Embedded Message Name"="", "Protobuf Index"=2, "MessageElementType"=enum."StringValue", "Repeated"=FALSE, "Is in Oneof"=FALSE, "Oneof Container Name"=""}, {"Field Name"="selected_index", "Embedded Message Name"="", "Protobuf Index"=-1, "MessageElementType"=enum."Int32Value", "Repeated"=FALSE, "Is in Oneof"=TRUE, "Oneof Container Name"="niswitch_grpc_RelayControlRequest_relay_action_enum"}, {"Field Name"="relay_action", "Embedded Message Name"="niswitch_grpc_RelayAction", "Protobuf Index"=3, "MessageElementType"=enum."EnumValue", "Repeated"=FALSE, "Is in Oneof"=TRUE, "Oneof Container Name"="niswitch_grpc_RelayControlRequest_relay_action_enum"}, {"Field Name"="relay_action_raw", "Embedded Message Name"="", "Protobuf Index"=4, "MessageElementType"=enum."SInt32", "Repeated"=FALSE, "Is in Oneof"=TRUE, "Oneof Container Name"="niswitch_grpc_RelayControlRequest_relay_action_enum"}], "Has Oneof"=TRUE}, {"Version"=2, "Name"="niswitch_grpc_RelayControlResponse", "Type Url"="niswitch_grpc.RelayControlResponse", "Elements"=[{"Field Name"="status", "Embedded Message Name"="", "Protobuf Index"=1, "MessageElementType"=enum."Int32Value", "Repeated"=FALSE, "Is in Oneof"=FALSE, "Oneof Container Name"=""}], "Has Oneof"=FALSE}, {"Version"=2, "Name"="niswitch_grpc_ResetRequest", "Type Url"="niswitch_grpc.ResetRequest", "Elements"=[{"Field Name"="vi", "Embedded Message Name"="nidevice_grpc_Session", "Protobuf Index"=1, "MessageElementType"=enum."MessageValue", "Repeated"=FALSE, "Is in Oneof"=FALSE, "Oneof Container Name"=""}], "Has Oneof"=FALSE}, {"Version"=2, "Name"="niswitch_grpc_ResetResponse", "Type Url"="niswitch_grpc.ResetResponse", "Elements"=[{"Field Name"="status", "Embedded Message Name"="", "Protobuf Index"=1, "MessageElementType"=enum."Int32Value", "Repeated"=FALSE, "Is in Oneof"=FALSE, "Oneof Container Name"=""}], "Has Oneof"=FALSE}, {"Version"=2, "Name"="niswitch_grpc_ResetInterchangeCheckRequest", "Type Url"="niswitch_grpc.ResetInterchangeCheckRequest", "Elements"=[{"Field Name"="vi", "Embedded Message Name"="nidevice_grpc_Session", "Protobuf Index"=1, "MessageElementType"=enum."MessageValue", "Repeated"=FALSE, "Is in Oneof"=FALSE, "Oneof Container Name"=""}], "Has Oneof"=FALSE}, {"Version"=2, "Name"="niswitch_grpc_ResetInterchangeCheckResponse", "Type Url"="niswitch_grpc.ResetInterchangeCheckResponse", "Elements"=[{"Field Name"="status", "Embedded Message Name"="", "Protobuf Index"=1, "MessageElementType"=enum."Int32Value", "Repeated"=FALSE, "Is in Oneof"=FALSE, "Oneof Container Name"=""}], "Has Oneof"=FALSE}, {"Version"=2, "Name"="niswitch_grpc_ResetWithDefaultsRequest", "Type Url"="niswitch_grpc.ResetWithDefaultsRequest", "Elements"=[{"Field Name"="vi", "Embedded Message Name"="nidevice_grpc_Session", "Protobuf Index"=1, "MessageElementType"=enum."MessageValue", "Repeated"=FALSE, "Is in Oneof"=FALSE, "Oneof Container Name"=""}], "Has Oneof"=FALSE}, {"Version"=2, "Name"="niswitch_grpc_ResetWithDefaultsResponse", "Type Url"="niswitch_grpc.ResetWithDefaultsResponse", "Elements"=[{"Field Name"="status", "Embedded Message Name"="", "Protobuf Index"=1, "MessageElementType"=enum."Int32Value", "Repeated"=FALSE, "Is in Oneof"=FALSE, "Oneof Container Name"=""}], "Has Oneof"=FALSE}, {"Version"=2, "Name"="niswitch_grpc_RevisionQueryRequest", "Type Url"="niswitch_grpc.RevisionQueryRequest", "Elements"=[{"Field Name"="vi", "Embedded Message Name"="nidevice_grpc_Session", "Protobuf Index"=1, "MessageElementType"=enum."MessageValue", "Repeated"=FALSE, "Is in Oneof"=FALSE, "Oneof Container Name"=""}], "Has Oneof"=FALSE}, {"Version"=2, "Name"="niswitch_grpc_RevisionQueryResponse", "Type Url"="niswitch_grpc.RevisionQueryResponse", "Elements"=[{"Field Name"="status", "Embedded Message Name"="", "Protobuf Index"=1, "MessageElementType"=enum."Int32Value", "Repeated"=FALSE, "Is in Oneof"=FALSE, "Oneof Container Name"=""}, {"Field Name"="instrument_driver_revision", "Embedded Message Name"="", "Protobuf Index"=2, "MessageElementType"=enum."StringValue", "Repeated"=FALSE, "Is in Oneof"=FALSE, "Oneof Container Name"=""}, {"Field Name"="firmware_revision", "Embedded Message Name"="", "Protobuf Index"=3, "MessageElementType"=enum."StringValue", "Repeated"=FALSE, "Is in Oneof"=FALSE, "Oneof Container Name"=""}], "Has Oneof"=FALSE}, {"Version"=2, "Name"="niswitch_grpc_RouteScanAdvancedOutputRequest", "Type Url"="niswitch_grpc.RouteScanAdvancedOutputRequest", "Elements"=[{"Field Name"="vi", "Embedded Message Name"="nidevice_grpc_Session", "Protobuf Index"=1, "MessageElementType"=enum."MessageValue", "Repeated"=FALSE, "Is in Oneof"=FALSE, "Oneof Container Name"=""}, {"Field Name"="selected_index", "Embedded Message Name"="", "Protobuf Index"=-1, "MessageElementType"=enum."Int32Value", "Repeated"=FALSE, "Is in Oneof"=TRUE, "Oneof Container Name"="niswitch_grpc_RouteScanAdvancedOutputRequest_scan_advanced_output_connector_enum"}, {"Field Name"="scan_advanced_output_connector", "Embedded Message Name"="niswitch_grpc_ScanAdvancedOutput", "Protobuf Index"=2, "MessageElementType"=enum."EnumValue", "Repeated"=FALSE, "Is in Oneof"=TRUE, "Oneof Container Name"="niswitch_grpc_RouteScanAdvancedOutputRequest_scan_advanced_output_connector_enum"}, {"Field Name"="scan_advanced_output_connector_raw", "Embedded Message Name"="", "Protobuf Index"=3, "MessageElementType"=enum."SInt32", "Repeated"=FALSE, "Is in Oneof"=TRUE, "Oneof Container Name"="niswitch_grpc_RouteScanAdvancedOutputRequest_scan_advanced_output_connector_enum"}, {"Field Name"="selected_index", "Embedded Message Name"="", "Protobuf Index"=-1, "MessageElementType"=enum."Int32Value", "Repeated"=FALSE, "Is in Oneof"=TRUE, "Oneof Container Name"="niswitch_grpc_RouteScanAdvancedOutputRequest_scan_advanced_output_bus_line_enum"}, {"Field Name"="scan_advanced_output_bus_line", "Embedded Message Name"="niswitch_grpc_ScanAdvancedOutput", "Protobuf Index"=4, "MessageElementType"=enum."EnumValue", "Repeated"=FALSE, "Is in Oneof"=TRUE, "Oneof Container Name"="niswitch_grpc_RouteScanAdvancedOutputRequest_scan_advanced_output_bus_line_enum"}, {"Field Name"="scan_advanced_output_bus_line_raw", "Embedded Message Name"="", "Protobuf Index"=5, "MessageElementType"=enum."SInt32", "Repeated"=FALSE, "Is in Oneof"=TRUE, "Oneof Container Name"="niswitch_grpc_RouteScanAdvancedOutputRequest_scan_advanced_output_bus_line_enum"}, {"Field Name"="invert", "Embedded Message Name"="", "Protobuf Index"=6, "MessageElementType"=enum."BoolValue", "Repeated"=FALSE, "Is in Oneof"=FALSE, "Oneof Container Name"=""}], "Has Oneof"=TRUE}, {"Version"=2, "Name"="niswitch_grpc_RouteScanAdvancedOutputResponse", "Type Url"="niswitch_grpc.RouteScanAdvancedOutputResponse", "Elements"=[{"Field Name"="status", "Embedded Message Name"="", "Protobuf Index"=1, "MessageElementType"=enum."Int32Value", "Repeated"=FALSE, "Is in Oneof"=FALSE, "Oneof Container Name"=""}], "Has Oneof"=FALSE}, {"Version"=2, "Name"="niswitch_grpc_RouteTriggerInputRequest", "Type Url"="niswitch_grpc.RouteTriggerInputRequest", "Elements"=[{"Field Name"="vi", "Embedded Message Name"="nidevice_grpc_Session", "Protobuf Index"=1, "MessageElementType"=enum."MessageValue", "Repeated"=FALSE, "Is in Oneof"=FALSE, "Oneof Container Name"=""}, {"Field Name"="selected_index", "Embedded Message Name"="", "Protobuf Index"=-1, "MessageElementType"=enum."Int32Value", "Repeated"=FALSE, "Is in Oneof"=TRUE, "Oneof Container Name"="niswitch_grpc_RouteTriggerInputRequest_trigger_input_connector_enum"}, {"Field Name"="trigger_input_connector", "Embedded Message Name"="niswitch_grpc_TriggerInput", "Protobuf Index"=2, "MessageElementType"=enum."EnumValue", "Repeated"=FALSE, "Is in Oneof"=TRUE, "Oneof Container Name"="niswitch_grpc_RouteTriggerInputRequest_trigger_input_connector_enum"}, {"Field Name"="trigger_input_connector_raw", "Embedded Message Name"="", "Protobuf Index"=3, "MessageElementType"=enum."SInt32", "Repeated"=FALSE, "Is in Oneof"=TRUE, "Oneof Container Name"="niswitch_grpc_RouteTriggerInputRequest_trigger_input_connector_enum"}, {"Field Name"="selected_index", "Embedded Message Name"="", "Protobuf Index"=-1, "MessageElementType"=enum."Int32Value", "Repeated"=FALSE, "Is in Oneof"=TRUE, "Oneof Container Name"="niswitch_grpc_RouteTriggerInputRequest_trigger_input_bus_line_enum"}, {"Field Name"="trigger_input_bus_line", "Embedded Message Name"="niswitch_grpc_TriggerInput", "Protobuf Index"=4, "MessageElementType"=enum."EnumValue", "Repeated"=FALSE, "Is in Oneof"=TRUE, "Oneof Container Name"="niswitch_grpc_RouteTriggerInputRequest_trigger_input_bus_line_enum"}, {"Field Name"="trigger_input_bus_line_raw", "Embedded Message Name"="", "Protobuf Index"=5, "MessageElementType"=enum."SInt32", "Repeated"=FALSE, "Is in Oneof"=TRUE, "Oneof Container Name"="niswitch_grpc_RouteTriggerInputRequest_trigger_input_bus_line_enum"}, {"Field Name"="invert", "Embedded Message Name"="", "Protobuf Index"=6, "MessageElementType"=enum."BoolValue", "Repeated"=FALSE, "Is in Oneof"=FALSE, "Oneof Container Name"=""}], "Has Oneof"=TRUE}, {"Version"=2, "Name"="niswitch_grpc_RouteTriggerInputResponse", "Type Url"="niswitch_grpc.RouteTriggerInputResponse", "Elements"=[{"Field Name"="status", "Embedded Message Name"="", "Protobuf Index"=1, "MessageElementType"=enum."Int32Value", "Repeated"=FALSE, "Is in Oneof"=FALSE, "Oneof Container Name"=""}], "Has Oneof"=FALSE}, {"Version"=2, "Name"="niswitch_grpc_ScanRequest", "Type Url"="niswitch_grpc.ScanRequest", "Elements"=[{"Field Name"="vi", "Embedded Message Name"="nidevice_grpc_Session", "Protobuf Index"=1, "MessageElementType"=enum."MessageValue", "Repeated"=FALSE, "Is in Oneof"=FALSE, "Oneof Container Name"=""}, {"Field Name"="scanlist", "Embedded Message Name"="", "Protobuf Index"=2, "MessageElementType"=enum."StringValue", "Repeated"=FALSE, "Is in Oneof"=FALSE, "Oneof Container Name"=""}, {"Field Name"="selected_index", "Embedded Message Name"="", "Protobuf Index"=-1, "MessageElementType"=enum."Int32Value", "Repeated"=FALSE, "Is in Oneof"=TRUE, "Oneof Container Name"="niswitch_grpc_ScanRequest_initiation_enum"}, {"Field Name"="initiation", "Embedded Message Name"="niswitch_grpc_HandshakingInitiation", "Protobuf Index"=3, "MessageElementType"=enum."EnumValue", "Repeated"=FALSE, "Is in Oneof"=TRUE, "Oneof Container Name"="niswitch_grpc_ScanRequest_initiation_enum"}, {"Field Name"="initiation_raw", "Embedded Message Name"="", "Protobuf Index"=4, "MessageElementType"=enum."SInt32", "Repeated"=FALSE, "Is in Oneof"=TRUE, "Oneof Container Name"="niswitch_grpc_ScanRequest_initiation_enum"}], "Has Oneof"=TRUE}, {"Version"=2, "Name"="niswitch_grpc_ScanResponse", "Type Url"="niswitch_grpc.ScanResponse", "Elements"=[{"Field Name"="status", "Embedded Message Name"="", "Protobuf Index"=1, "MessageElementType"=enum."Int32Value", "Repeated"=FALSE, "Is in Oneof"=FALSE, "Oneof Container Name"=""}], "Has Oneof"=FALSE}, {"Version"=2, "Name"="niswitch_grpc_SelfTestRequest", "Type Url"="niswitch_grpc.SelfTestRequest", "Elements"=[{"Field Name"="vi", "Embedded Message Name"="nidevice_grpc_Session", "Protobuf Index"=1, "MessageElementType"=enum."MessageValue", "Repeated"=FALSE, "Is in Oneof"=FALSE, "Oneof Container Name"=""}], "Has Oneof"=FALSE}, {"Version"=2, "Name"="niswitch_grpc_SelfTestResponse", "Type Url"="niswitch_grpc.SelfTestResponse", "Elements"=[{"Field Name"="status", "Embedded Message Name"="", "Protobuf Index"=1, "MessageElementType"=enum."Int32Value", "Repeated"=FALSE, "Is in Oneof"=FALSE, "Oneof Container Name"=""}, {"Field Name"="self_test_result", "Embedded Message Name"="", "Protobuf Index"=2, "MessageElementType"=enum."SInt32", "Repeated"=FALSE, "Is in Oneof"=FALSE, "Oneof Container Name"=""}, {"Field Name"="self_test_message", "Embedded Message Name"="", "Protobuf Index"=3, "MessageElementType"=enum."StringValue", "Repeated"=FALSE, "Is in Oneof"=FALSE, "Oneof Container Name"=""}], "Has Oneof"=FALSE}, {"Version"=2, "Name"="niswitch_grpc_SendSoftwareTriggerRequest", "Type Url"="niswitch_grpc.SendSoftwareTriggerRequest", "Elements"=[{"Field Name"="vi", "Embedded Message Name"="nidevice_grpc_Session", "Protobuf Index"=1, "MessageElementType"=enum."MessageValue", "Repeated"=FALSE, "Is in Oneof"=FALSE, "Oneof Container Name"=""}], "Has Oneof"=FALSE}, {"Version"=2, "Name"="niswitch_grpc_SendSoftwareTriggerResponse", "Type Url"="niswitch_grpc.SendSoftwareTriggerResponse", "Elements"=[{"Field Name"="status", "Embedded Message Name"="", "Protobuf Index"=1, "MessageElementType"=enum."Int32Value", "Repeated"=FALSE, "Is in Oneof"=FALSE, "Oneof Container Name"=""}], "Has Oneof"=FALSE}, {"Version"=2, "Name"="niswitch_grpc_SetAttributeViBooleanRequest", "Type Url"="niswitch_grpc.SetAttributeViBooleanRequest", "Elements"=[{"Field Name"="vi", "Embedded Message Name"="nidevice_grpc_Session", "Protobuf Index"=1, "MessageElementType"=enum."MessageValue", "Repeated"=FALSE, "Is in Oneof"=FALSE, "Oneof Container Name"=""}, {"Field Name"="channel_name", "Embedded Message Name"="", "Protobuf Index"=2, "MessageElementType"=enum."StringValue", "Repeated"=FALSE, "Is in Oneof"=FALSE, "Oneof Container Name"=""}, {"Field Name"="attribute_id", "Embedded Message Name"="niswitch_grpc_NiSwitchAttribute", "Protobuf Index"=3, "MessageElementType"=enum."EnumValue", "Repeated"=FALSE, "Is in Oneof"=FALSE, "Oneof Container Name"=""}, {"Field Name"="attribute_value", "Embedded Message Name"="", "Protobuf Index"=4, "MessageElementType"=enum."BoolValue", "Repeated"=FALSE, "Is in Oneof"=FALSE, "Oneof Container Name"=""}], "Has Oneof"=FALSE}, {"Version"=2, "Name"="niswitch_grpc_SetAttributeViBooleanResponse", "Type Url"="niswitch_grpc.SetAttributeViBooleanResponse", "Elements"=[{"Field Name"="status", "Embedded Message Name"="", "Protobuf Index"=1, "MessageElementType"=enum."Int32Value", "Repeated"=FALSE, "Is in Oneof"=FALSE, "Oneof Container Name"=""}], "Has Oneof"=FALSE}, {"Version"=2, "Name"="niswitch_grpc_SetAttributeViInt32Request", "Type Url"="niswitch_grpc.SetAttributeViInt32Request", "Elements"=[{"Field Name"="vi", "Embedded Message Name"="nidevice_grpc_Session", "Protobuf Index"=1, "MessageElementType"=enum."MessageValue", "Repeated"=FALSE, "Is in Oneof"=FALSE, "Oneof Container Name"=""}, {"Field Name"="channel_name", "Embedded Message Name"="", "Protobuf Index"=2, "MessageElementType"=enum."StringValue", "Repeated"=FALSE, "Is in Oneof"=FALSE, "Oneof Container Name"=""}, {"Field Name"="attribute_id", "Embedded Message Name"="niswitch_grpc_NiSwitchAttribute", "Protobuf Index"=3, "MessageElementType"=enum."EnumValue", "Repeated"=FALSE, "Is in Oneof"=FALSE, "Oneof Container Name"=""}, {"Field Name"="selected_index", "Embedded Message Name"="", "Protobuf Index"=-1, "MessageElementType"=enum."Int32Value", "Repeated"=FALSE, "Is in Oneof"=TRUE, "Oneof Container Name"="niswitch_grpc_SetAttributeViInt32Request_attribute_value_enum"}, {"Field Name"="attribute_value_raw", "Embedded Message Name"="", "Protobuf Index"=4, "MessageElementType"=enum."SInt32", "Repeated"=FALSE, "Is in Oneof"=TRUE, "Oneof Container Name"="niswitch_grpc_SetAttributeViInt32Request_attribute_value_enum"}, {"Field Name"="attribute_value", "Embedded Message Name"="niswitch_grpc_NiSwitchInt32AttributeValues", "Protobuf Index"=5, "MessageElementType"=enum."EnumValue", "Repeated"=FALSE, "Is in Oneof"=TRUE, "Oneof Container Name"="niswitch_grpc_SetAttributeViInt32Request_attribute_value_enum"}], "Has Oneof"=TRUE}, {"Version"=2, "Name"="niswitch_grpc_SetAttributeViInt32Response", "Type Url"="niswitch_grpc.SetAttributeViInt32Response", "Elements"=[{"Field Name"="status", "Embedded Message Name"="", "Protobuf Index"=1, "MessageElementType"=enum."Int32Value", "Repeated"=FALSE, "Is in Oneof"=FALSE, "Oneof Container Name"=""}], "Has Oneof"=FALSE}, {"Version"=2, "Name"="niswitch_grpc_SetAttributeViReal64Request", "Type Url"="niswitch_grpc.SetAttributeViReal64Request", "Elements"=[{"Field Name"="vi", "Embedded Message Name"="nidevice_grpc_Session", "Protobuf Index"=1, "MessageElementType"=enum."MessageValue", "Repeated"=FALSE, "Is in Oneof"=FALSE, "Oneof Container Name"=""}, {"Field Name"="channel_name", "Embedded Message Name"="", "Protobuf Index"=2, "MessageElementType"=enum."StringValue", "Repeated"=FALSE, "Is in Oneof"=FALSE, "Oneof Container Name"=""}, {"Field Name"="attribute_id", "Embedded Message Name"="niswitch_grpc_NiSwitchAttribute", "Protobuf Index"=3, "MessageElementType"=enum."EnumValue", "Repeated"=FALSE, "Is in Oneof"=FALSE, "Oneof Container Name"=""}, {"Field Name"="attribute_value_raw", "Embedded Message Name"="", "Protobuf Index"=4, "MessageElementType"=enum."DoubleValue", "Repeated"=FALSE, "Is in Oneof"=FALSE, "Oneof Container Name"=""}], "Has Oneof"=FALSE}, {"Version"=2, "Name"="niswitch_grpc_SetAttributeViReal64Response", "Type Url"="niswitch_grpc.SetAttributeViReal64Response", "Elements"=[{"Field Name"="status", "Embedded Message Name"="", "Protobuf Index"=1, "MessageElementType"=enum."Int32Value", "Repeated"=FALSE, "Is in Oneof"=FALSE, "Oneof Container Name"=""}], "Has Oneof"=FALSE}, {"Version"=2, "Name"="niswitch_grpc_SetAttributeViSessionRequest", "Type Url"="niswitch_grpc.SetAttributeViSessionRequest", "Elements"=[{"Field Name"="vi", "Embedded Message Name"="nidevice_grpc_Session", "Protobuf Index"=1, "MessageElementType"=enum."MessageValue", "Repeated"=FALSE, "Is in Oneof"=FALSE, "Oneof Container Name"=""}, {"Field Name"="channel_name", "Embedded Message Name"="", "Protobuf Index"=2, "MessageElementType"=enum."StringValue", "Repeated"=FALSE, "Is in Oneof"=FALSE, "Oneof Container Name"=""}, {"Field Name"="attribute_id", "Embedded Message Name"="niswitch_grpc_NiSwitchAttribute", "Protobuf Index"=3, "MessageElementType"=enum."EnumValue", "Repeated"=FALSE, "Is in Oneof"=FALSE, "Oneof Container Name"=""}, {"Field Name"="attribute_value", "Embedded Message Name"="nidevice_grpc_Session", "Protobuf Index"=4, "MessageElementType"=enum."MessageValue", "Repeated"=FALSE, "Is in Oneof"=FALSE, "Oneof Container Name"=""}], "Has Oneof"=FALSE}, {"Version"=2, "Name"="niswitch_grpc_SetAttributeViSessionResponse", "Type Url"="niswitch_grpc.SetAttributeViSessionResponse", "Elements"=[{"Field Name"="status", "Embedded Message Name"="", "Protobuf Index"=1, "MessageElementType"=enum."Int32Value", "Repeated"=FALSE, "Is in Oneof"=FALSE, "Oneof Container Name"=""}], "Has Oneof"=FALSE}, {"Version"=2, "Name"="niswitch_grpc_SetAttributeViStringRequest", "Type Url"="niswitch_grpc.SetAttributeViStringRequest", "Elements"=[{"Field Name"="vi", "Embedded Message Name"="nidevice_grpc_Session", "Protobuf Index"=1, "MessageElementType"=enum."MessageValue", "Repeated"=FALSE, "Is in Oneof"=FALSE, "Oneof Container Name"=""}, {"Field Name"="channel_name", "Embedded Message Name"="", "Protobuf Index"=2, "MessageElementType"=enum."StringValue", "Repeated"=FALSE, "Is in Oneof"=FALSE, "Oneof Container Name"=""}, {"Field Name"="attribute_id", "Embedded Message Name"="niswitch_grpc_NiSwitchAttribute", "Protobuf Index"=3, "MessageElementType"=enum."EnumValue", "Repeated"=FALSE, "Is in Oneof"=FALSE, "Oneof Container Name"=""}, {"Field Name"="attribute_value_raw", "Embedded Message Name"="", "Protobuf Index"=4, "MessageElementType"=enum."StringValue", "Repeated"=FALSE, "Is in Oneof"=FALSE, "Oneof Container Name"=""}], "Has Oneof"=FALSE}, {"Version"=2, "Name"="niswitch_grpc_SetAttributeViStringResponse", "Type Url"="niswitch_grpc.SetAttributeViStringResponse", "Elements"=[{"Field Name"="status", "Embedded Message Name"="", "Protobuf Index"=1, "MessageElementType"=enum."Int32Value", "Repeated"=FALSE, "Is in Oneof"=FALSE, "Oneof Container Name"=""}], "Has Oneof"=FALSE}, {"Version"=2, "Name"="niswitch_grpc_SetContinuousScanRequest", "Type Url"="niswitch_grpc.SetContinuousScanRequest", "Elements"=[{"Field Name"="vi", "Embedded Message Name"="nidevice_grpc_Session", "Protobuf Index"=1, "MessageElementType"=enum."MessageValue", "Repeated"=FALSE, "Is in Oneof"=FALSE, "Oneof Container Name"=""}, {"Field Name"="continuous_scan", "Embedded Message Name"="", "Protobuf Index"=2, "MessageElementType"=enum."BoolValue", "Repeated"=FALSE, "Is in Oneof"=FALSE, "Oneof Container Name"=""}], "Has Oneof"=FALSE}, {"Version"=2, "Name"="niswitch_grpc_SetContinuousScanResponse", "Type Url"="niswitch_grpc.SetContinuousScanResponse", "Elements"=[{"Field Name"="status", "Embedded Message Name"="", "Protobuf Index"=1, "MessageElementType"=enum."Int32Value", "Repeated"=FALSE, "Is in Oneof"=FALSE, "Oneof Container Name"=""}], "Has Oneof"=FALSE}, {"Version"=2, "Name"="niswitch_grpc_SetPathRequest", "Type Url"="niswitch_grpc.SetPathRequest", "Elements"=[{"Field Name"="vi", "Embedded Message Name"="nidevice_grpc_Session", "Protobuf Index"=1, "MessageElementType"=enum."MessageValue", "Repeated"=FALSE, "Is in Oneof"=FALSE, "Oneof Container Name"=""}, {"Field Name"="path_list", "Embedded Message Name"="", "Protobuf Index"=2, "MessageElementType"=enum."StringValue", "Repeated"=FALSE, "Is in Oneof"=FALSE, "Oneof Container Name"=""}], "Has Oneof"=FALSE}, {"Version"=2, "Name"="niswitch_grpc_SetPathResponse", "Type Url"="niswitch_grpc.SetPathResponse", "Elements"=[{"Field Name"="status", "Embedded Message Name"="", "Protobuf Index"=1, "MessageElementType"=enum."Int32Value", "Repeated"=FALSE, "Is in Oneof"=FALSE, "Oneof Container Name"=""}], "Has Oneof"=FALSE}, {"Version"=2, "Name"="niswitch_grpc_WaitForDebounceRequest", "Type Url"="niswitch_grpc.WaitForDebounceRequest", "Elements"=[{"Field Name"="vi", "Embedded Message Name"="nidevice_grpc_Session", "Protobuf Index"=1, "MessageElementType"=enum."MessageValue", "Repeated"=FALSE, "Is in Oneof"=FALSE, "Oneof Container Name"=""}, {"Field Name"="maximum_time_ms", "Embedded Message Name"="", "Protobuf Index"=2, "MessageElementType"=enum."SInt32", "Repeated"=FALSE, "Is in Oneof"=FALSE, "Oneof Container Name"=""}], "Has Oneof"=FALSE}, {"Version"=2, "Name"="niswitch_grpc_WaitForDebounceResponse", "Type Url"="niswitch_grpc.WaitForDebounceResponse", "Elements"=[{"Field Name"="status", "Embedded Message Name"="", "Protobuf Index"=1, "MessageElementType"=enum."Int32Value", "Repeated"=FALSE, "Is in Oneof"=FALSE, "Oneof Container Name"=""}], "Has Oneof"=FALSE}, {"Version"=2, "Name"="niswitch_grpc_WaitForScanCompleteRequest", "Type Url"="niswitch_grpc.WaitForScanCompleteRequest", "Elements"=[{"Field Name"="vi", "Embedded Message Name"="nidevice_grpc_Session", "Protobuf Index"=1, "MessageElementType"=enum."MessageValue", "Repeated"=FALSE, "Is in Oneof"=FALSE, "Oneof Container Name"=""}, {"Field Name"="maximum_time_ms", "Embedded Message Name"="", "Protobuf Index"=2, "MessageElementType"=enum."SInt32", "Repeated"=FALSE, "Is in Oneof"=FALSE, "Oneof Container Name"=""}], "Has Oneof"=FALSE}, {"Version"=2, "Name"="niswitch_grpc_WaitForScanCompleteResponse", "Type Url"="niswitch_grpc.WaitForScanCompleteResponse", "Elements"=[{"Field Name"="status", "Embedded Message Name"="", "Protobuf Index"=1, "MessageElementType"=enum."Int32Value", "Repeated"=FALSE, "Is in Oneof"=FALSE, "Oneof Container Name"=""}], "Has Oneof"=FALSE}, {"Version"=2, "Name"="nidevice_grpc_Session", "Type Url"="nidevice_grpc.Session", "Elements"=[{"Field Name"="name", "Embedded Message Name"="", "Protobuf Index"=1, "MessageElementType"=enum."StringValue", "Repeated"=FALSE, "Is in Oneof"=FALSE, "Oneof Container Name"=""}], "Has Oneof"=FALSE}]  # Messages MetaData
      n2 = call <vilib>:"Register Message Metadata.vi"("error in"=w10, "Messages"=w11, "gRPCid in"=w9) -> ("error out"=w7:errorcluster, "gRPCid out"=w8:T1)  [unwired: 7 in]
      n3 = call <vilib>:"Register Enum Metadata.vi"("error in"=w7, "Enum Metadata"=w5, "gRPCid in"=w8) -> ("error out"=w6:errorcluster)  [unwired: 7 in, 1 out]
    }
    frame Error {
    }
  }
  "error out" <- w4
  "gRPC ID Out" <- w1
